vi "Do_Every_minute.vi"(1 "Ch Names":string[](array[string]), 2 "Values":dbl[](array[numeric]) format="%.2f") -> (0 "Scan Comments":string)   [LabVIEW 2022 SP3]
uses:
  Anemometry/Anemometry Sub Vis/Controls/In_Range.ctl
  ADAM Client/Sub VIs/ADAM Controls/Update_scan_value.ctl
  ADAM Client/Sub VIs/Channel_State_Control.ctl
  ADAM Client/Sub VIs/ADAM Controls/Traverse_Level_State.ctl
  Anemometry/Anemometry Sub Vis/Globals/EnFlo_Tunnel_Global.vi
  Anemometry/Anemometry Sub Vis/Globals/Gas_management_global.vi
  ADAM_Global.vi
panel:
  in  "Kp":dbl=50.0 format="%#_13g"
  in  "Deadband Delta T":dbl=0.002 format="%#_13g"
  out "Max Delta T":dbl(graph)
  in  "Manual Control of Lamps":bool
  out "Power":dbl[][](graph)=[[0.00729, 0.18153463174730816, 0.17352738437348433, 1.6752433719500537, 8.231465735195274, 17.570357598383207, 23.099772817121426, 25.58386930448374, 25.31727725753219, 24.28926231541072, 18.717383219374323, 10.355253339797807, 2.7760273383248344, 0.3109897541921306, 0.08276881403435009, 0.06197], [0.04411, 0.1361526368018142, 0.04039202183336771, 1.5611636795339547, 8.176972694107874, 17.32000974741714, 24.257541358764026, 25.949153465972987, 26.01802540761648, 25.060373307424115, 18.284750328365213, 8.689831176707928, 2.642937641487066, 0.43219350072447926, -0.019957690739617468, 0.07351], [0.05478, 0.03446320268089581, 0.2086595806581808, 1.6919212249796047, 6.580368005180591, 14.333585185483123, 21.06810094963999, 23.709254571137723, 24.04768940379576, 21.01660820522005, 13.60443428327954, 6.2766496258038735, 1.7988963349022484, 0.2952877651784204, 0.05436788410934033, 0.1022], [0.04013, 0.06419557464541133, 0.2035068586120256, 1.3118741659450193, 4.7061387064566835, 9.009825946069038, 12.927700276268434, 17.003135081884164, 16.83885730812343, 12.902263313363814, 8.246161922417906, 4.035269404379355, 1.329605659745338, 0.24574055091433544, 0.012829784119986217, 0.08755], [0.04404, 0.022691144295571734, 0.19102098261858932, 0.8525411026079828, 2.2353542219792946, 3.966676465246214, 6.305347763088489, 8.17672908183636, 7.7348668140659, 5.703994479070454, 3.8329088824353237, 1.9256956625267279, 0.6611488869641811, 0.20508248283573002, 0.10119553469307395, 0.08441]]
  out "Temperature":dbl[][](graph)=[[0.00729, 0.18153463174730816, 0.17352738437348433, 1.6752433719500537, 8.231465735195274, 17.570357598383207, 23.099772817121426, 25.58386930448374, 25.31727725753219, 24.28926231541072, 18.717383219374323, 10.355253339797807, 2.7760273383248344, 0.3109897541921306, 0.08276881403435009, 0.06197], [0.04411, 0.1361526368018142, 0.04039202183336771, 1.5611636795339547, 8.176972694107874, 17.32000974741714, 24.257541358764026, 25.949153465972987, 26.01802540761648, 25.060373307424115, 18.284750328365213, 8.689831176707928, 2.642937641487066, 0.43219350072447926, -0.019957690739617468, 0.07351], [0.05478, 0.03446320268089581, 0.2086595806581808, 1.6919212249796047, 6.580368005180591, 14.333585185483123, 21.06810094963999, 23.709254571137723, 24.04768940379576, 21.01660820522005, 13.60443428327954, 6.2766496258038735, 1.7988963349022484, 0.2952877651784204, 0.05436788410934033, 0.1022], [0.04013, 0.06419557464541133, 0.2035068586120256, 1.3118741659450193, 4.7061387064566835, 9.009825946069038, 12.927700276268434, 17.003135081884164, 16.83885730812343, 12.902263313363814, 8.246161922417906, 4.035269404379355, 1.329605659745338, 0.24574055091433544, 0.012829784119986217, 0.08755], [0.04404, 0.022691144295571734, 0.19102098261858932, 0.8525411026079828, 2.2353542219792946, 3.966676465246214, 6.305347763088489, 8.17672908183636, 7.7348668140659, 5.703994479070454, 3.8329088824353237, 1.9256956625267279, 0.6611488869641811, 0.20508248283573002, 0.10119553469307395, 0.08441]]
  in  "Kp Lamps":dbl=50.0 format="%#_13g"
  in  "Averaging time in Seconds":dbl=200.0 format="%#_13g"
  in  "Disable Sending email to estates regarding Chilled water Temp":bool=TRUE
  in  "Max K Factor":dbl=16.0
  # "Control Parameters"
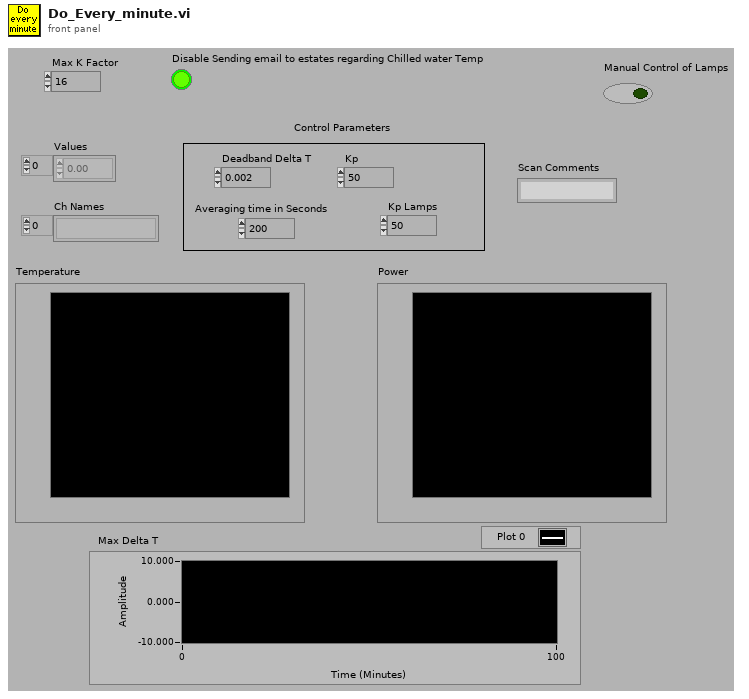
[diagram p1: front panel]
types:
  T1 = typedef "In_Range.ctl" = enum16{"%", "±", "% & ±"}
  T2 = typedef "Update_scan_value.ctl" = cluster{"Channel Name":string, "New Value":dbl, "!Auto_Off":bool}
  T3 = enum16{"Append to Global", "Read Global then Clear"}
  T4 = typedef "Channel_State_Control.ctl" = enum16{"Channel Name", "Channel Name Starts with", "Main Address"}
  T5 = typedef "Traverse_Level_State.ctl" = enum16{"Running", "Complete"}
  T6 = typedef "Ch_description_ADAM.ctl" = cluster{"Ch Name":string, "Type":T7, "Function":T8, "Ch State":T9, "Calibration type":T10, "A":dbl, "B":dbl, "C":dbl, "D":dbl, "Comments":string, "Address":T11, "String":string, "Duty":u16}
  T7 = typedef "Module_type_ADAM.ctl" = string
  T8 = typedef "Function_ADAM.ctl" = enum16{"Analogue Input", "Digital Input", "Event counter", "Event rate", "Analogue Output", "Digital Output", "Relay Output"}
  T9 = typedef "Channel_State.ctl" = enum16{"On", "Off", "Always On", "Always Off"}
  T10 = typedef "Calib_type_ADAM.ctl" = string
  T11 = typedef "Address.ctl" = cluster{"Main":i32, "Ch.":i32, "Sub":i32, "Port Name":string}
  T12 = cluster{"Bus Bar":string, "Connected Items":string[]}
  T13 = cluster{"Ch Name":string, "subarray":string[], "subarray":dbl[], i32, i32}
  T14 = typedef "Client_State_Cluster.ctl" = cluster{"Client Name":string, "Traverse level State":T5, "People to Email":string[], "Next Contact Time":dbl}
  T15 = cluster{"second":i32, "minute":i32, "hour":i32, "day of month":i32, "month":i32, "year":i32, "day of week":i32, "day of year":i32, "is DST":i32}
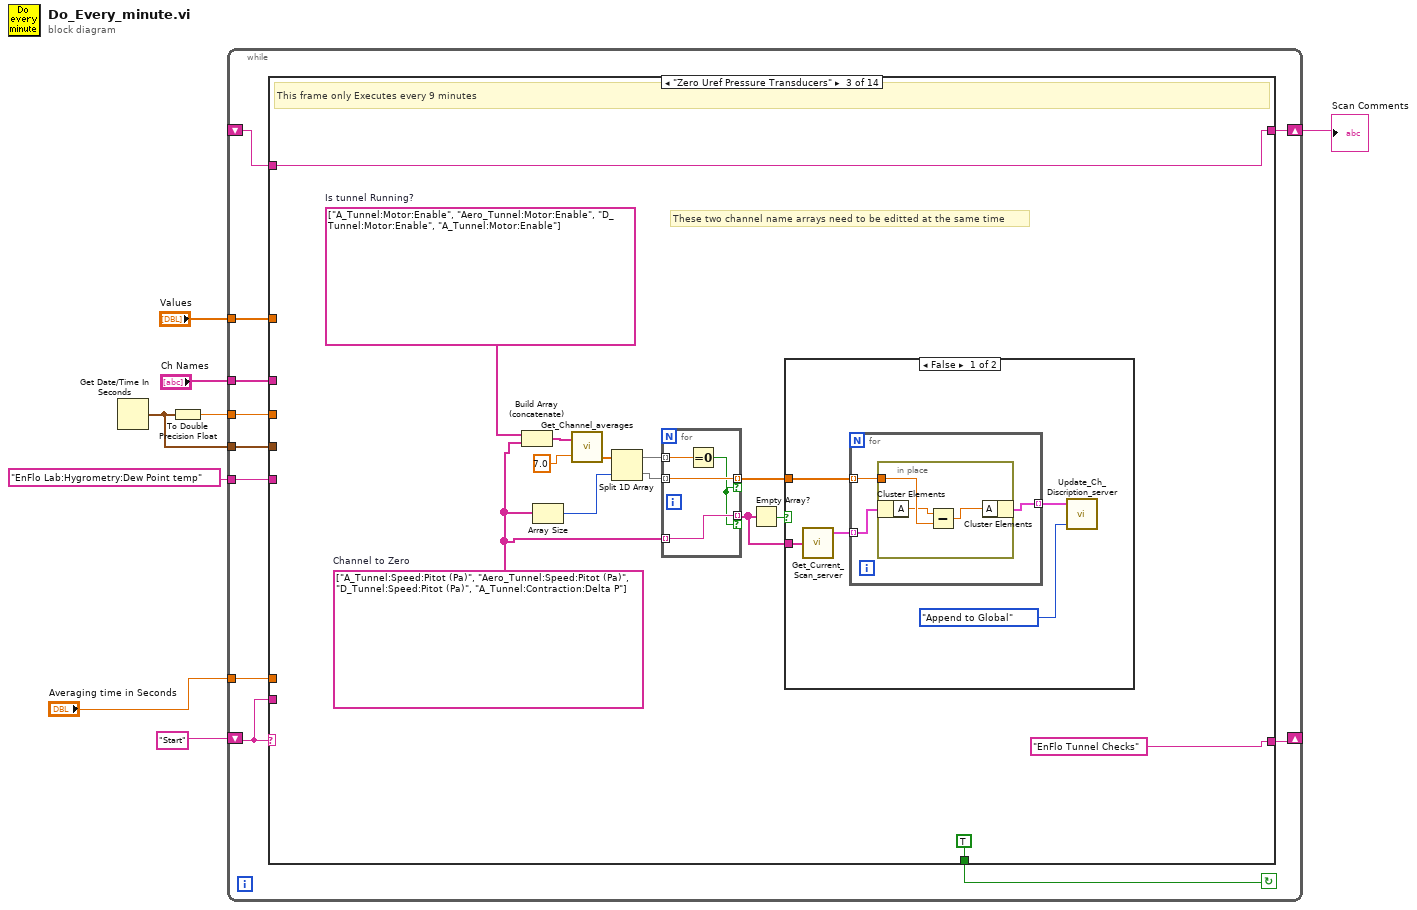
[diagram p0: block diagram]
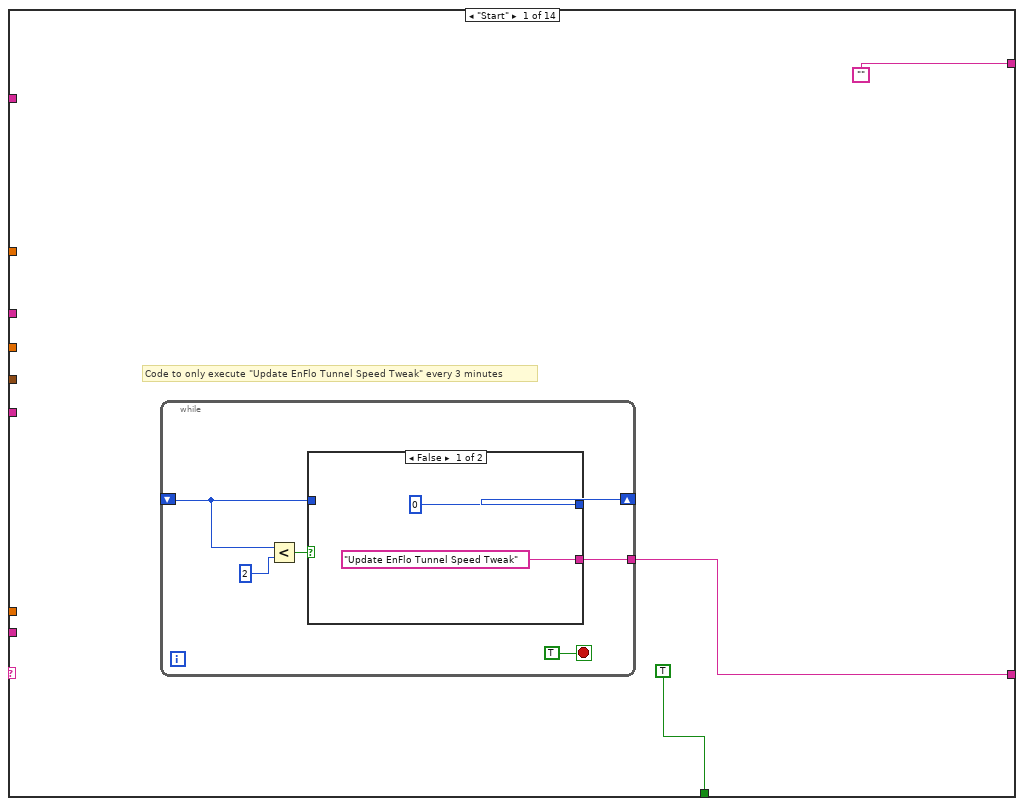
[diagram p2: hidden frame]
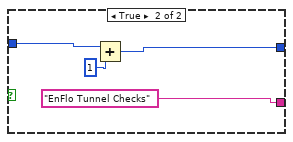
[diagram p3: hidden frame]
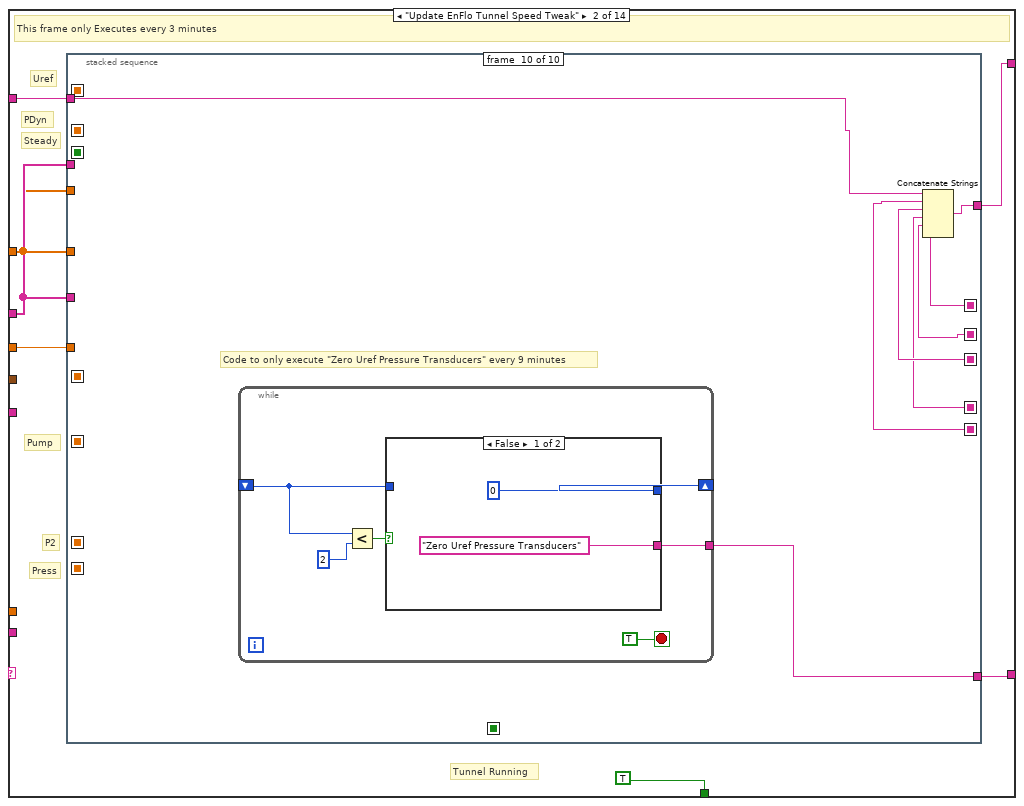
[diagram p4: hidden frame]
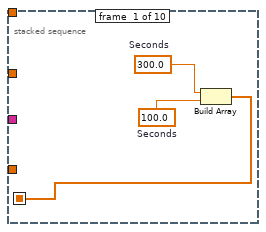
[diagram p5: hidden frame]
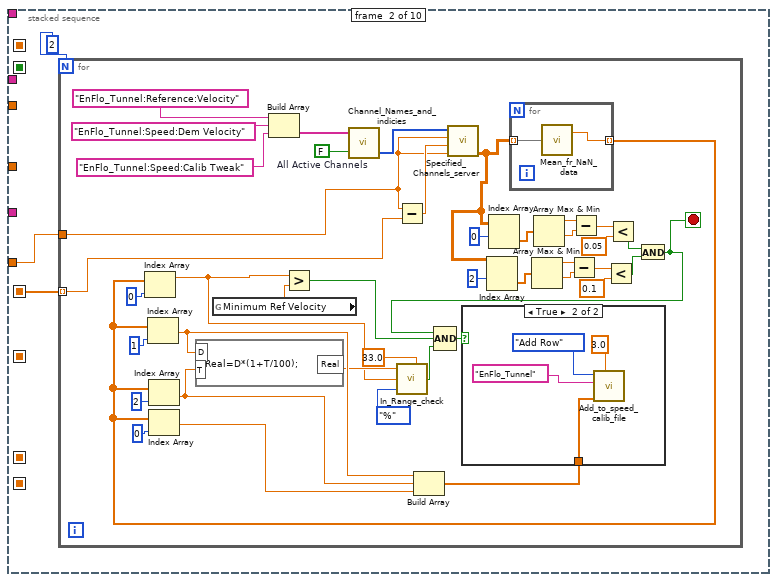
[diagram p6: hidden frame]
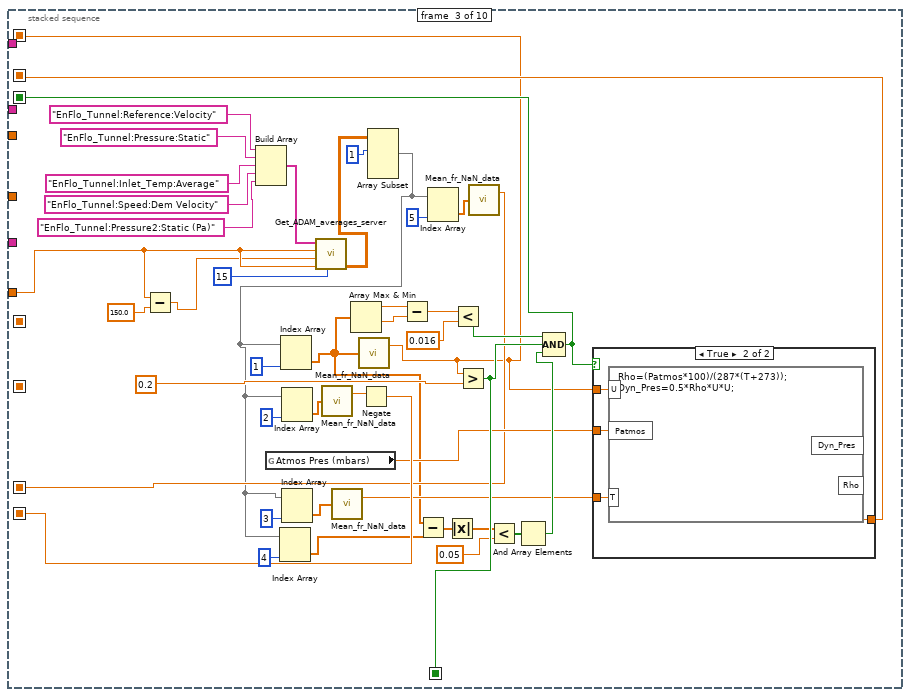
[diagram p8: hidden frame]
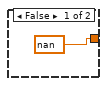
[diagram p9: hidden frame]
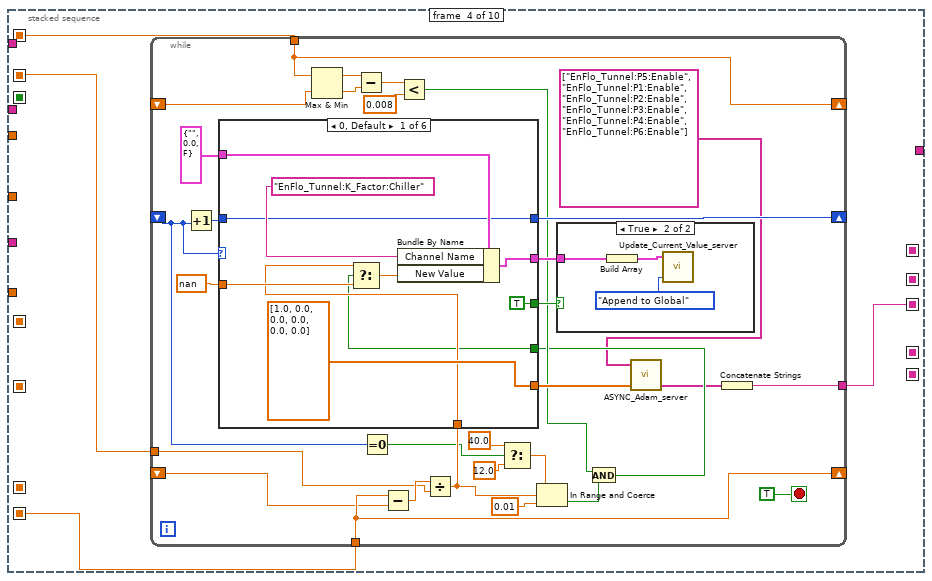
[diagram p10: hidden frame]
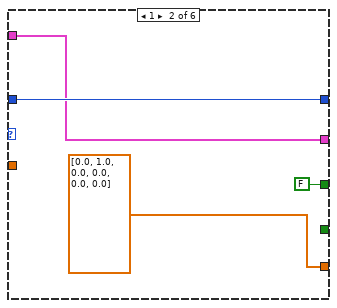
[diagram p12: hidden frame]
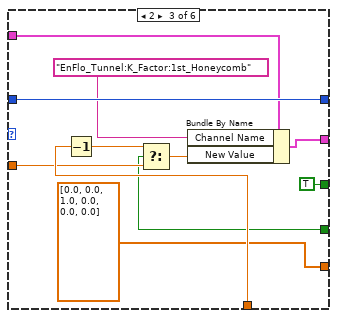
[diagram p13: hidden frame]
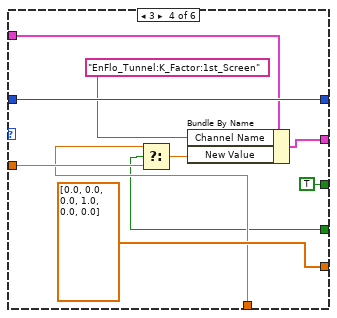
[diagram p14: hidden frame]
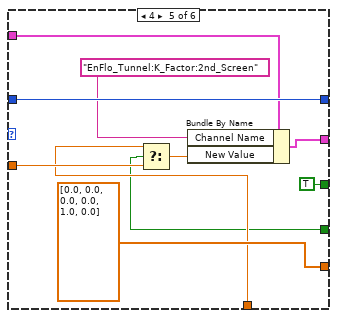
[diagram p15: hidden frame]
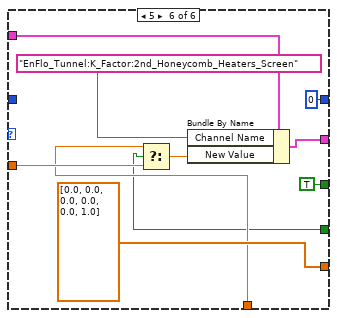
[diagram p16: hidden frame]
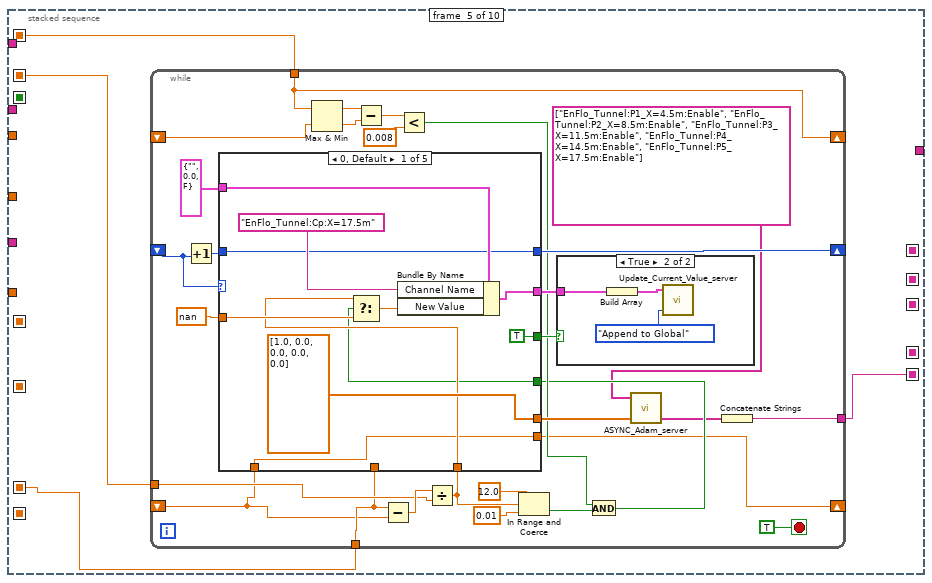
[diagram p17: hidden frame]
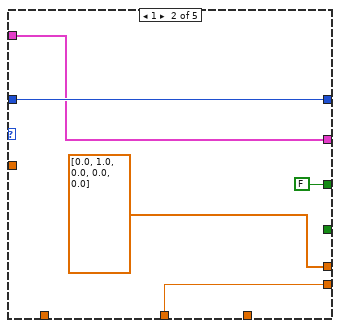
[diagram p19: hidden frame]
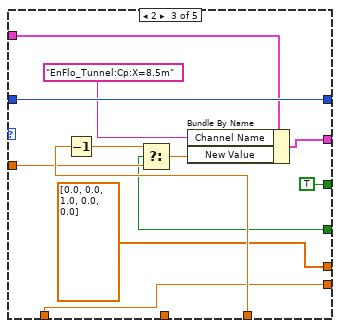
[diagram p20: hidden frame]
diagram:
  n1 = Get Date/Time In Seconds() -> (seconds since 1Jan1904=w4:timestamp)
  n2 = To Double Precision Float(number=w4) -> (double precision float=w5:dbl)
  n3 = while {
    tunnel: "EnFlo Lab:Hygrometry:Dew Point temp" -> [w15]
    tunnel: "Values" -> [w17]
    tunnel: "Ch Names" -> [w18]
    shift-left: "Start" -> [w12]
    shift-right: [w16] -> _
    tunnel: w5 -> [w14]
    tunnel: w4 -> [w13]
    tunnel: "Averaging time in Seconds" -> [w11]
    shift-right: [w10] -> w1
    shift-left: _ -> [w9]
    stop <- w19 continue-if-true
    n4 = case shown="\"Zero Uref Pressure Transducers\"" w12 {
      tunnel: [TRUE TRUE TRUE TRUE TRUE TRUE TRUE TRUE TRUE TRUE TRUE TRUE FALSE FALSE] -> w19
      tunnel: w18 -> [_ w37 _ w530 w725 _ _ _ w1013 w1040 w1076 w1116 w1128 _]
      tunnel: w17 -> [_ w36 _ w531 w726 _ _ _ w1014 w1041 w1077 w1117 w1127 _]
      tunnel: [w21 w35 "EnFlo Tunnel Checks" w529 w724 w953 "Lab Temp Control" "Is Dew point meter Alive?" w1017 w1028 "More checks" "End" "End" "End"] -> w16
      tunnel: w15 -> [_ _ _ _ _ _ _ _ w1012 _ _ _ _ _]
      tunnel: w14 -> [_ w40 _ w528 w728 _ _ w991 _ _ _ _ w1126 _]
      tunnel: w13 -> [_ _ _ _ _ _ _ _ _ _ _ _ w1129 _]
      tunnel: w12 -> [_ _ _ _ _ _ _ _ _ _ _ _ _ w1196]
      tunnel: w11 -> [_ _ _ w527 w727 _ _ _ _ _ _ _ _ _]
      tunnel: ["" w38 w497 w525 w722 w951 w966 w990 w994 w1026 w1065 w1112 w1122 w1193] -> w10
      tunnel: w9 -> [_ w39 w497 w526 w723 w951 w966 w990 w996 w1027 w1066 w1113 w1123 w1193]
      frame "Start" {
        # "Code to only execute \"Update EnFlo Tunnel Speed Tweak\" every 3 minutes"
        n5 = while {
          shift-right: [w25] -> _
          shift-left: _ -> [w23]
          tunnel: [w24] -> w21
          stop <- TRUE stop-if-true
          n6 = Less?(x=w23, y=2) -> (x < y?=w26:bool)
          n7 = case shown="False" w26 {
            tunnel: [0 w32] -> w25
            tunnel: ["Update EnFlo Tunnel Speed Tweak" "EnFlo Tunnel Checks"] -> w24
            tunnel: w23 -> [_ w33]
            frame False {
            }
            frame True {
              n8 = Add(x=w33, y=1) -> (x+y=w32:i32)
            }
          }
        }
      }
      frame "Update EnFlo Tunnel Speed Tweak" {
        # "P2"
        # "Pump"
        # "Tunnel Running"
        # "PDyn"
        # "Steady"
        # "Press"
        # "Uref"
        # "This frame only Executes every 3 minutes"
        n9 = stacked-sequence {
          seq-local: [w42 _ _ _ _ _ _ _ _ _] -> [_ w46 _ _ _ _ _ _ _ _]
          seq-local: [_ _ w99 _ _ _ _ _ _ _] -> [_ _ _ w145 w240 _ _ _ _ _]
          seq-local: [_ _ w123 _ _ _ _ _ _ _] -> [_ _ _ w147 _ _ _ _ _ _]
          seq-local: [_ _ w121 _ _ _ _ _ _ _] -> [_ _ _ _ _ _ _ _ _ _]
          seq-local: [_ _ w124 _ _ _ _ _ _ _] -> [_ _ _ w146 w238 _ _ _ _ _]
          seq-local: [_ _ w120 _ _ _ _ _ _ _] -> [_ _ _ _ _ _ _ w384 _ _]
          seq-local: [_ _ _ w144 _ _ _ _ _ _] -> [_ _ _ _ _ _ _ _ _ w482]
          seq-local: [_ _ _ _ _ w324 _ _ _ _] -> [_ _ _ _ _ _ w332 _ _ _]
          seq-local: [_ _ _ _ _ w323 _ _ _ _] -> [_ _ _ _ _ _ _ _ _ w480]
          seq-local: [_ _ _ _ _ _ w328 _ _ _] -> [_ _ _ _ _ _ _ _ _ w479]
          seq-local: [_ _ _ _ _ _ _ w383 _ _] -> [_ _ _ _ _ _ _ _ _ w478]
          seq-local: [_ _ w105 _ _ _ _ _ _ _] -> [_ _ _ _ w237 _ _ _ _ _]
          seq-local: [_ _ _ _ w239 _ _ _ _ _] -> [_ _ _ _ _ _ _ _ _ w477]
          tunnel: w37 -> [_ _ _ _ _ w326 w329 _ _ _]
          tunnel: w36 -> [_ _ _ _ _ w327 w330 _ _ _]
          tunnel: w40 -> [_ w45 w138 _ _ _ _ w382 _ _]
          tunnel: w39 -> [_ _ _ _ _ _ _ _ _ w483]
          tunnel: [_ _ _ _ _ _ _ _ _ w481] -> w38
          tunnel: w37 -> [_ _ _ _ _ _ _ _ _ _]
          tunnel: w36 -> [_ _ _ _ _ _ _ _ _ _]
          tunnel: [_ _ _ _ _ _ _ _ _ w476] -> w35
          frame #0 {
            w43 = 100.0  # Seconds
            w44 = 300.0  # Seconds
            n10 = Build Array(w44, w43) -> (w42:dbl[])
          }
          frame #1 {
            n11 = for {
              N: 2 -> [_]
              tunnel: w45 -> [w51]
              tunnel: w46 -> [w50] mode=indexing
              stop <- w49 stop-if-true
              w81 = FALSE  # All Active Channels
              n12 = global read "EnFlo_Tunnel_Global.vi" "Minimum Ref Velocity"() -> (w48:dbl)
              n13 = Build Array("EnFlo_Tunnel:Reference:Velocity", "EnFlo_Tunnel:Speed:Dem Velocity", "EnFlo_Tunnel:Speed:Calib Tweak") -> (w79:string[])
              n14 = call "Channel_Names_and_indicies.vi"("All Active Channels"=w81, "Desired Ch Names"=w79) -> ("Indicies"=w80:i32[])  [unwired: 1 out]
              n15 = Subtract(x=w51, y=w50) -> (x-y=w78:dbl)
              n16 = call "Specified_Channels_server.vi"("End time"=w51, "Start time"=w78, "Clients time"=w51, "Requested channels"=w80) -> ("Output array"=w61:dbl[][])  [unwired: 1 in, 4 out]
              n17 = Index Array(array=w61, index (row)=2 ("Index")) -> (element=w63:dbl[])  [unwired: 1 in]
              n18 = Index Array(array=w61, index (row)=0 ("Index")) -> (element=w76:dbl[])  [unwired: 1 in]
              n19 = for {
                tunnel: w61 -> [w91] mode=indexing
                tunnel: [w90] -> w69 mode=indexing
                n20 = call "Mean_fr_NaN_data.vi"("Data"=w91) -> ("Mean value"=w90:dbl)  [unwired: 1 out]
              }
              n21 = Index Array(array=w69, index=0) -> (element=w55:dbl)
              n22 = Index Array(array=w69, index=1) -> (element=w57:dbl)
              n23 = Index Array(array=w69, index=2) -> (element=w58:dbl)
              n24 = Index Array(array=w69, index=0) -> (element=w68:dbl)
              n25 = formula code="Real=D*(1+T/100);"("D"=w57, "T"=w58) -> ("Real"=w56:dbl)
              n26 = Greater?(x=w55, y=w48) -> (0:w84:bool)
              n27 = call "In_Range_check.vi"("%"=33.0, "Mode"=In_Range."%", "Value"=w55, "Setpoint"=w56) -> ("In Range"=w52:bool)  [unwired: 1 in, 2 out]
              n28 = Build Array(w57, w58, w68) -> (w83:dbl[])
              n29 = Array Max & Min(array=w63) -> (max value=w64:dbl, min value=w65:dbl)  [unwired: 2 out]
              n30 = Array Max & Min(array=w76) -> (max value=w75:dbl, min value=w74:dbl)  [unwired: 2 out]
              n31 = Subtract(x=w64, y=w65) -> (x-y=w66:dbl)
              n32 = Subtract(x=w75, y=w74) -> (x-y=w73:dbl)
              n33 = Less?(x=w66, y=0.1) -> (x < y?=w60:bool)
              n34 = Less?(x=w73, y=0.05) -> (x < y?=w59:bool)
              n35 = And(x=w59, y=w60) -> (x .and. y?=w49:bool)
              n36 = Compound Arithmetic op=AND(w49, w84, w52) -> (w82:bool)
              n37 = case shown="True" w82 {
                tunnel: w83 -> [_ w94]
                frame False {
                }
                frame True {
                  n38 = call "Add_to_speed_calib_file.vi"("Max Velocity"=3.0, "New Row"=w94, "Rig Name"="EnFlo_Tunnel" ("y"), "Mode"=enum16{"Add Row", "Get Error Value"}."Add Row") -> ()  [unwired: 2 in, 2 out]
                }
              }
            }
          }
          frame #2 {
            n39 = Subtract(x=w138, y=150.0) -> (x-y=w136:dbl)
            n40 = Build Array("EnFlo_Tunnel:Reference:Velocity", "EnFlo_Tunnel:Pressure:Static", "EnFlo_Tunnel:Inlet_Temp:Average", "EnFlo_Tunnel:Speed:Dem Velocity", "EnFlo_Tunnel:Pressure2:Static (Pa)") -> (w135:string[])
            n41 = global read "Gas_management_global.vi" "Atmos Pres (mbars)"() -> (w107:dbl)
            n42 = call "Get_ADAM_averages_server.vi"("No of averages"=15, "End time"=w138, "Start time"=w136, "Clients time"=w138, "ADAM Ch Names"=w135) -> ("DBL values"=w98:dbl[][])  [unwired: 1 in, 4 out]
            n43 = Array Subset(array=w98, index (row)=1 ("index")) -> (w96:dbl[][])  [unwired: 3 in]
            n44 = Index Array(array=w96, index (col)=4 ("disabled index (col)")) -> (element=w113:dbl[])  [unwired: 1 in]
            n45 = Index Array(array=w96, index (col)=1 ("disabled index (col)")) -> (element=w100:dbl[])  [unwired: 1 in]
            n46 = Index Array(array=w96, index (col)=2 ("disabled index (col)")) -> (element=w102:dbl[])  [unwired: 1 in]
            n47 = Index Array(array=w96, index (col)=3 ("disabled index (col)")) -> (element=w104:dbl[])  [unwired: 1 in]
            n48 = call "Mean_fr_NaN_data.vi"("Data"=w102) -> ("Mean value"=w101:dbl)  [unwired: 1 out]
            n49 = call "Mean_fr_NaN_data.vi"("Data"=w104) -> ("Mean value"=w103:dbl)  [unwired: 1 out]
            n50 = Array Max & Min(array=w100) -> (max value=w130:dbl, min value=w131:dbl)  [unwired: 2 out]
            n51 = call "Mean_fr_NaN_data.vi"("Data"=w100) -> ("Mean value"=w99:dbl)  [unwired: 1 out]
            n52 = Negate(x=w101) -> (-x=w123:dbl)
            n53 = Subtract(x=w130, y=w131) -> (x-y=w132:dbl)
            n54 = Subtract(x=w100, y=w113) -> (x-y=w116:dbl[])
            n55 = Index Array(array=w96, index (col)=5 ("disabled index (col)")) -> (element=w106:dbl[])  [unwired: 1 in]
            n56 = Absolute Value(x=w116) -> (abs(x)=w115:dbl[])
            n57 = Less?(x=w132, y=0.016) -> (x < y?=w122:bool)
            n58 = Greater?(x=w99, y=0.2) -> (0:w120:bool)
            n59 = call "Mean_fr_NaN_data.vi"("Data"=w106) -> ("Mean value"=w105:dbl)  [unwired: 1 out]
            n60 = Less?(x=w115, y=0.05) -> (x < y?=w112:bool[])
            n61 = And Array Elements(Boolean array=w112) -> (logical AND=w111:bool)
            n62 = Compound Arithmetic op=AND(w122, w120, w111) -> (w121:bool)
            n63 = case shown="True" w121 {
              tunnel: w103 -> [_ w143]
              tunnel: w107 -> [_ w142]
              tunnel: w99 -> [_ w141]
              tunnel: [nan w140] -> w124
              frame False {
              }
              frame True {
                n64 = formula code="Rho=(Patmos*100)/(287*(T+273));\nDyn_Pres=0.5*Rho*U*U;"("Patmos"=w142, "T"=w143, "U"=w141) -> ("Dyn_Pres"=w140:dbl)  [unwired: 1 out]
              }
            }
          }
          frame #3 {
            n65 = while {
              shift-right: [w177] -> _
              shift-left: _ -> [w152]
              shift-right: [w174] -> _
              shift-left: _ -> [w173]
              tunnel: w147 -> [w174]
              tunnel: w146 -> [w171]
              shift-right: [w170] -> _
              shift-left: _ -> [w169]
              tunnel: w145 -> [w170]
              tunnel: [w154] -> w144
              stop <- TRUE stop-if-true
              n66 = Increment(x=w152) -> (x+1=w176:i32)
              n67 = Max & Min(x=w170, y=w169) -> (max(x,y)=w168:dbl, min(x,y)=w167:dbl)
              n68 = Subtract(x=w168, y=w167) -> (x-y=w166:dbl)
              n69 = Equal To 0?(x=w152) -> (x = 0?=w150:bool)
              n70 = Subtract(x=w174, y=w173) -> (x-y=w172:dbl)
              n71 = Less?(x=w166, y=0.008) -> (x < y?=w157:bool)
              n72 = Divide(x=w172, y=w171) -> (x/y=w160:dbl)
              n73 = Select(t=40.0 ("upper limit"), s=w150, f=12.0) -> (s? t:f=w149:dbl)
              n74 = In Range and Coerce(upper limit=w149, x=w160, lower limit=0.01) -> (In Range?=w158:bool)  [unwired: 1 out]
              n75 = And(x=w157, y=w158) -> (x .and. y?=w156:bool)
              n76 = case shown="0, Default" w152 {
                tunnel: [w184 w195 w206 w216 w226 0] -> w177
                tunnel: w176 -> [w184 w195 w206 w216 w226 _]
                tunnel: T2 {"Channel Name"="", "New Value"=0.0, "!Auto_Off"=FALSE} ("Update Scan Value Cluster") -> [w191 w194 w205 w215 w225 w236]
                tunnel: w160 -> [w185 _ w203 w209 w219 w230]
                tunnel: [w189 w194 w202 w213 w223 w234] -> w164
                tunnel: nan -> [w188 _ w200 w212 w222 w233]
                tunnel: [dbl[] [1.0, 0.0, 0.0, 0.0, 0.0, 0.0] ("Values") dbl[] [0.0, 1.0, 0.0, 0.0, 0.0, 0.0] ("Values") dbl[] [0.0, 0.0, 1.0, 0.0, 0.0, 0.0] ("Values") dbl[] [0.0, 0.0, 0.0, 1.0, 0.0, 0.0] ("Values") dbl[] [0.0, 0.0, 0.0, 0.0, 1.0, 0.0] ("Values") dbl[] [0.0, 0.0, 0.0, 0.0, 0.0, 1.0] ("Values")] -> w162
                tunnel: [TRUE FALSE TRUE TRUE TRUE TRUE] -> w161
                tunnel: w156 -> [w182 _ w196 w207 w217 w227]
                frame 0, Default {
                  n77 = Select(t=w185, s=w182, f=w188) -> (s? t:f=w187:dbl)
                  n78 = Bundle By Name(cluster=w191, "Channel Name"="EnFlo_Tunnel:K_Factor:Chiller", "New Value"=w187) -> (w189:T2)
                }
                frame 1 {
                }
                frame 2 {
                  n79 = Decrement(x=w203) -> (x-1=w201:dbl)
                  n80 = Select(t=w201, s=w196, f=w200) -> (s? t:f=w199:dbl)
                  n81 = Bundle By Name(cluster=w205, "Channel Name"="EnFlo_Tunnel:K_Factor:1st_Honeycomb", "New Value"=w199) -> (w202:T2)
                }
                frame 3 {
                  n82 = Select(t=w209, s=w207, f=w212) -> (s? t:f=w211:dbl)
                  n83 = Bundle By Name(cluster=w215, "Channel Name"="EnFlo_Tunnel:K_Factor:1st_Screen", "New Value"=w211) -> (w213:T2)
                }
                frame 4 {
                  n84 = Select(t=w219, s=w217, f=w222) -> (s? t:f=w221:dbl)
                  n85 = Bundle By Name(cluster=w225, "Channel Name"="EnFlo_Tunnel:K_Factor:2nd_Screen", "New Value"=w221) -> (w223:T2)
                }
                frame 5 {
                  n86 = Select(t=w230, s=w227, f=w233) -> (s? t:f=w232:dbl)
                  n87 = Bundle By Name(cluster=w236, "Channel Name"="EnFlo_Tunnel:K_Factor:2nd_Honeycomb_Heaters_Screen", "New Value"=w232) -> (w234:T2)
                }
              }
              n88 = case shown="True" w161 {
                tunnel: w164 -> [_ w179]
                frame False {
                }
                frame True {
                  n89 = Build Array(w179) -> (w180:T2[])
                  n90 = call "Update_Current_Value_server.vi"("Mode"=T3."Append to Global", "Update array in"=w180) -> ()  [unwired: 1 in, 1 out]
                }
              }
              n91 = call "ASYNC_Adam_server.vi"("Values"=w162, "Channel Names"=string[] ["EnFlo_Tunnel:P5:Enable", "EnFlo_Tunnel:P1:Enable", "EnFlo_Tunnel:P2:Enable", "EnFlo_Tunnel:P3:Enable", "EnFlo_Tunnel:P4:Enable", "EnFlo_Tunnel:P6:Enable"]) -> ("Scan Comments"=w155:string[])  [unwired: 1 in, 2 out]
              n92 = Concatenate Strings(w155) -> (w154:string)
            }
          }
          frame #4 {
            n93 = while {
              shift-right: [w268] -> _
              shift-left: _ -> [w266]
              shift-right: [w244] -> _
              shift-left: _ -> [w242]
              tunnel: w237 -> [w243]
              tunnel: w238 -> [w263]
              shift-right: [w262] -> _
              shift-left: _ -> [w261]
              tunnel: w240 -> [w262]
              tunnel: [w245] -> w239
              stop <- TRUE stop-if-true
              n94 = Increment(x=w266) -> (x+1=w267:i32)
              n95 = Max & Min(x=w262, y=w261) -> (max(x,y)=w260:dbl, min(x,y)=w259:dbl)
              n96 = Subtract(x=w260, y=w259) -> (x-y=w258:dbl)
              n97 = Subtract(x=w243, y=w242) -> (x-y=w264:dbl)
              n98 = Less?(x=w258, y=0.008) -> (x < y?=w248:bool)
              n99 = Divide(x=w264, y=w263) -> (x/y=w252:dbl)
              n100 = In Range and Coerce(upper limit=12.0, x=w252, lower limit=0.01) -> (In Range?=w249:bool)  [unwired: 1 out]
              n101 = And(x=w248, y=w249) -> (x .and. y?=w247:bool)
              n102 = case shown="0, Default" w266 {
                tunnel: [w276 w288 w300 w311 0] -> w268
                tunnel: w267 -> [w276 w288 w300 w311 _]
                tunnel: T2 {"Channel Name"="", "New Value"=0.0, "!Auto_Off"=FALSE} ("Update Scan Value Cluster") -> [w283 w287 w299 w310 w322]
                tunnel: w252 -> [w277 _ w297 w304 w316]
                tunnel: [w281 w287 w296 w308 w320] -> w256
                tunnel: nan -> [w280 _ w294 w307 w319]
                tunnel: [dbl[] [1.0, 0.0, 0.0, 0.0, 0.0] ("Values") dbl[] [0.0, 1.0, 0.0, 0.0, 0.0] ("Values") dbl[] [0.0, 0.0, 1.0, 0.0, 0.0] ("Values") dbl[] [0.0, 0.0, 0.0, 1.0, 0.0] ("Values") dbl[] [0.0, 0.0, 0.0, 0.0, 1.0] ("Values")] -> w254
                tunnel: [TRUE FALSE TRUE TRUE TRUE] -> w253
                tunnel: w247 -> [w274 _ w290 w302 w313]
                tunnel: [w273 w284 w289 w301 w312] -> w244
                tunnel: w243 -> [_ w284 _ _ _]
                tunnel: w242 -> [w273 _ w289 w301 w312]
                frame 0, Default {
                  n103 = Select(t=w277, s=w274, f=w280) -> (s? t:f=w279:dbl)
                  n104 = Bundle By Name(cluster=w283, "Channel Name"="EnFlo_Tunnel:Cp:X=17.5m", "New Value"=w279) -> (w281:T2)
                }
                frame 1 {
                }
                frame 2 {
                  n105 = Decrement(x=w297) -> (x-1=w295:dbl)
                  n106 = Select(t=w295, s=w290, f=w294) -> (s? t:f=w293:dbl)
                  n107 = Bundle By Name(cluster=w299, "Channel Name"="EnFlo_Tunnel:Cp:X=8.5m", "New Value"=w293) -> (w296:T2)
                }
                frame 3 {
                  n108 = Select(t=w304, s=w302, f=w307) -> (s? t:f=w306:dbl)
                  n109 = Bundle By Name(cluster=w310, "Channel Name"="EnFlo_Tunnel:Cp:X=11.5m", "New Value"=w306) -> (w308:T2)
                }
                frame 4 {
                  n110 = Select(t=w316, s=w313, f=w319) -> (s? t:f=w318:dbl)
                  n111 = Bundle By Name(cluster=w322, "Channel Name"="EnFlo_Tunnel:Cp:X=14.5m", "New Value"=w318) -> (w320:T2)
                }
              }
              n112 = case shown="True" w253 {
                tunnel: w256 -> [_ w270]
                frame False {
                }
                frame True {
                  n113 = Build Array(w270) -> (w271:T2[])
                  n114 = call "Update_Current_Value_server.vi"("Mode"=T3."Append to Global", "Update array in"=w271) -> ()  [unwired: 1 in, 1 out]
                }
              }
              n115 = call "ASYNC_Adam_server.vi"("Values"=w254, "Channel Names"=string[] ["EnFlo_Tunnel:P1_X=4.5m:Enable", "EnFlo_Tunnel:P2_X=8.5m:Enable", "EnFlo_Tunnel:P3_X=11.5m:Enable", "EnFlo_Tunnel:P4_X=14.5m:Enable", "EnFlo_Tunnel:P5_X=17.5m:Enable"]) -> ("Scan Comments"=w246:string[])  [unwired: 1 in, 2 out]
              n116 = Concatenate Strings(w246) -> (w245:string)
            }
          }
          frame #5 {
            n117 = call "Read_value_of_earlier_Ch.vi"("Desired Ch to Read"="EnFlo_Tunnel:Chiller_Pump:Running", "Ch names"=w326, "Present scan array"=w327) -> ("Value"=w324:dbl, "Scan comment"=w323:string)  [unwired: 1 in]
          }
          frame #6 {
            n118 = Greater?(x=w332, y=0.5) -> (0:w331:bool)
            n119 = case shown="True" w331 {
              tunnel: w330 -> [_ w355]
              tunnel: w329 -> [_ w354]
              tunnel: ["" w345] -> w328
              frame False {
              }
              frame True {
                w348 = errorcluster {"status"=FALSE, "code"=0, "source"=""} ("error in (no error)")
                w347 = string[] ["EnFlo_Tunnel:Power:Chiller_Pump_Exchanger", "EnFlo_Tunnel:Meas Power:Chiller_Pump_Exchanger", "EnFlo_Tunnel:Power:Chiller_Pump_Floor", "EnFlo_Tunnel:Meas Power:Chiller_Pump_Floor"]
                n120 = call "Read_Earlier_Channels.vi"("Present scan array"=w355, "Ch names"=w354, "Desired Channels"=w347) -> ("Scan comments"=w345:string, "Index 0"=w344:dbl, "Index 1"=w349:dbl, "Index 2"=w339:dbl, "Index 3"=w346:dbl)  [unwired: 1 out]
                n121 = feedback-in #1(w344) -> ()
                n122 = feedback #1() -> (w343:dbl)  [unwired: 1 in]
                n123 = Equal?(x=w343, y=w344) -> (x = y?=w342:bool)
                n124 = call "In_Range_check.vi"("±"=6.0, "Mode"=In_Range."±", "Value"=w346, "Setpoint"=w339) -> ("In Range"=w336:bool)  [unwired: 3 in]
                n125 = call "In_Range_check.vi"("±"=6.0, "Mode"=In_Range."±", "Value"=w349, "Setpoint"=w344) -> ("In Range"=w341:bool)  [unwired: 3 in]
                n126 = feedback #2() -> (w338:dbl)  [unwired: 1 in]
                n127 = feedback-in #2(w339) -> ()
                n128 = Compound Arithmetic op=AND(w342, invert w341) -> (w340:bool)
                n129 = Equal?(x=w339, y=w338) -> (x = y?=w337:bool)
                n130 = Compound Arithmetic op=AND(w337, invert w336) -> (w335:bool)
                n131 = case shown="True" w340 {
                  tunnel: w348 -> [_ _]
                  tunnel: w347 -> [_ w381]
                  tunnel: w344 -> [_ w378]
                  tunnel: w349 -> [_ w377]
                  frame False {
                  }
                  frame True {
                    n132 = Index Array(array=w381, index #1=0 ("index"), index #2=1 ("index")) -> (element #1=w370:string, element #2=w375:string)
                    n133 = Format Into String(format string="Warning\n%s=%.0f %s=%.0f", w370, w378, w375, w377) -> (resulting string=w373:string)  [unwired: 2 in, 1 out]
                    n134 = call "Fast_string_Replace.vi"("Replace match with:"=" ", "Input String"=w370, "matchThis"=":" ("regular expression")) -> ("Output String"=w369:string)  [unwired: 1 in, 1 out]
                    n135 = call "Server_Emails.vi"("Client Name Contains"="EnFlo_Tunnel", "Message"=w373, "Subject"=w369) -> ()  [unwired: 2 in, 3 out]
                  }
                }
                n136 = case shown="True" w335 {
                  tunnel: w348 -> [_ _]
                  tunnel: w347 -> [_ w368]
                  tunnel: w339 -> [_ w365]
                  tunnel: w346 -> [_ w364]
                  frame False {
                  }
                  frame True {
                    n137 = Index Array(array=w368, index #1=2 ("index"), index #2=3 ("index")) -> (element #1=w359:string, element #2=w362:string)
                    n138 = Format Into String(format string="Warning\n%s=%.0f %s=%.0f", w359, w365, w362, w364) -> (resulting string=w360:string)  [unwired: 2 in, 1 out]
                    n139 = call "Fast_string_Replace.vi"("Replace match with:"=" ", "Input String"=w359, "matchThis"=":" ("regular expression")) -> ("Output String"=w358:string)  [unwired: 1 in, 1 out]
                    n140 = call "Server_Emails.vi"("Client Name Contains"="EnFlo_Tunnel", "Message"=w360, "Subject"=w358) -> ()  [unwired: 2 in, 3 out]
                  }
                }
              }
            }
          }
          frame #7 {
            n141 = case shown="True" w384 {
              tunnel: w382 -> [_ w389]
              tunnel: ["" w390] -> w383
              tunnel: w382 -> [_ w387]
              tunnel: w382 -> [_ w386]
              frame False {
              }
              frame True {
                w391 = string[] ["EnFlo_Tunnel:Temp:Pre_Inlet_Y=1500_Z=450", "EnFlo_Tunnel:Temp:Pre_Inlet_Y=-1500_Z=450", "EnFlo_Tunnel:Temp:Pre_Inlet_Y=1000_Z=450", "EnFlo_Tunnel:Temp:Pre_Inlet_Y=-1000_Z=450", "EnFlo_Tunnel:Temp:Pre_Inlet_Y=500_Z=450"] ("Sub set")
                n142 = Subtract(x=w389, y=300.0 ("x-y")) -> (x-y=w403:dbl)
                n143 = call "Get_ADAM_averages_client.vi"("No of averages"=1, "End time"=w389, "Start time"=w403, "ADAM Ch Names"=w391) -> ("Messages"=w390:string, "DBL values"=w407:dbl[][])  [unwired: 3 in, 3 out]
                n144 = Index Array(array=w407, index (row)=1 ("disabled index (col)")) -> (element=w402:dbl[])  [unwired: 1 in]
                n145 = Array Subset(array=w402, index=1, length=5) -> (w400:dbl[])
                n146 = Array Max & Min(array=w400) -> (max value=w397:dbl, max index (indices)=w395:i32, min value=w399:dbl, min index (indices)=w396:i32)
                n147 = Subtract(x=w397, y=w399) -> (x-y=w392:dbl)
                n148 = Index Array(array=w391, index=w396) -> (element=w393:string)
                n149 = Greater Or Equal?(x=w392, y=0.3) -> (x >= y?=w388:bool)
                n150 = Index Array(array=w391, index=w395) -> (element=w394:string)
                n151 = case shown="True" w388 {
                  tunnel: w394 -> [_ w423]
                  tunnel: w393 -> [_ w422]
                  tunnel: w392 -> [_ w421]
                  tunnel: w387 -> [_ w413]
                  tunnel: w386 -> [_ w411]
                  frame False {
                  }
                  frame True {
                    n152 = Subtract(x=w413, y=1200.0) -> (x-y=w416:dbl)
                    n153 = call "Get_ADAM_averages_client.vi"("No of averages"=20, "End time"=w411, "Start time"=w416, "ADAM Ch Names"=string[] ["EnFlo_Tunnel:Reference:Velocity"]) -> ("DBL values"=w419:dbl[][])  [unwired: 3 in, 4 out]
                    n154 = global read "EnFlo_Tunnel_Global.vi" "Minimum Ref Velocity for taking Results"() -> (w417:dbl)
                    n155 = Index Array(array=w419, index (col)=1 ("disabled index (col)")) -> (element=w418:dbl[])  [unwired: 1 in]
                    n156 = Greater Or Equal?(x=w418, y=w417) -> (x >= y?=w420:bool[])
                    n157 = And Array Elements(Boolean array=w420) -> (logical AND=w409:bool)
                    n158 = case shown="True" w409 {
                      tunnel: w421 -> [_ w426]
                      tunnel: w422 -> [_ w425]
                      tunnel: w423 -> [_ w424]
                      frame False {
                      }
                      frame True {
                        n159 = Format Into String(format string="The %s is %.2f degC more than %s.\\n Check the inlet fans are operating correctly." ("Format String"), w424, w426, w425) -> (resulting string=w428:string)  [unwired: 2 in, 1 out]
                        n160 = call "Server_Emails.vi"("Client Name Contains"="EnFlo_Tunnel", "Message"=w428, "Subject"="Large Inlet Temperature Variation" ("Error Type")) -> ()  [unwired: 2 in, 3 out]
                      }
                    }
                  }
                }
              }
            }
          }
          frame #8 {
            w440 = "EnFlo_Tunnel:Motor:Enable"
            w443 = "A_Tunnel:Motor:Enable"
            w452 = "Aero_Tunnel:Motor:Enable"
            # "Turning off Tunnel Drives if not used for more than"
            n161 = Build Array("A_Tunnel:Speed:Dem Velocity", w443) -> (w450:string[])
            n162 = Build Array("EnFlo_Tunnel:Speed:Dem Velocity", w440) -> (w431:string[])
            n163 = Build Array (concatenate)("Aero_Tunnel:Speed:Dem Velocity", w452, w450, w431) -> (w458:string[])
            n164 = call "Get_Channel_averages.vi"("Desired Ch Names"=w458, "Averaging time (mins)"=20.0) -> ("number"=w432:dbl[])  [unwired: 1 in, 2 out]
            n165 = Index Array(array=w432, index #1=2 ("index"), index #2=3 ("index")) -> (element #1=w445:dbl, element #2=w444:dbl)
            n166 = Index Array(array=w432, index #1=4 ("index"), index #2=5 ("index")) -> (element #1=w438:dbl, element #2=w439:dbl)
            n167 = Index Array(array=w432) -> (element #1=w457:dbl, element #2=w456:dbl)  [unwired: 2 in]
            n168 = Equal To 0?(x=w445) -> (x = 0?=w447:bool)
            n169 = Greater Than 0?(x=w444) -> (x > 0?=w446:bool)
            n170 = Equal To 0?(x=w438) -> (x = 0?=w436:bool)
            n171 = Greater Than 0?(x=w439) -> (x > 0?=w437:bool)
            n172 = Equal To 0?(x=w457) -> (x = 0?=w454:bool)
            n173 = Greater Than 0?(x=w456) -> (x > 0?=w455:bool)
            n174 = And(x=w447, y=w446) -> (x .and. y?=w442:bool)
            n175 = case shown="True" w442 {
              tunnel: w443 -> [_ w471]
              frame False {
              }
              frame True {
                n176 = Build Array(w471) -> (w470:string[])
                n177 = Build Array(0.0) -> (w469:dbl[])
                n178 = call "ASYNC_Adam_server.vi"("Values"=w469, "Channel Names"=w470) -> ()  [unwired: 1 in, 3 out]
              }
            }
            n179 = And(x=w436, y=w437) -> (x .and. y?=w441:bool)
            n180 = case shown="True" w441 {
              tunnel: w440 -> [_ w467]
              frame False {
              }
              frame True {
                n181 = Build Array(w467) -> (w466:string[])
                n182 = Build Array(0.0) -> (w465:dbl[])
                n183 = call "ASYNC_Adam_server.vi"("Values"=w465, "Channel Names"=w466) -> ()  [unwired: 1 in, 3 out]
                n184 = call "Ch_Active_Control.vi"("Match"="EnFlo_Tunnel:Drive:In Standby", "Activate Channels?"=FALSE, "Control on"=Channel_State_Control."Channel Name") -> ()  [unwired: 1 in, 2 out]
              }
            }
            n185 = And(x=w454, y=w455) -> (x .and. y?=w453:bool)
            n186 = case shown="True" w453 {
              tunnel: w452 -> [_ w475]
              frame False {
              }
              frame True {
                n187 = Build Array(w475) -> (w474:string[])
                n188 = Build Array(0.0) -> (w473:dbl[])
                n189 = call "ASYNC_Adam_server.vi"("Values"=w473, "Channel Names"=w474) -> ()  [unwired: 1 in, 3 out]
              }
            }
          }
          frame #9 {
            # "Code to only execute \"Zero Uref Pressure Transducers\" every 9 minutes"
            n190 = while {
              shift-right: [w486] -> _
              shift-left: _ -> [w484]
              tunnel: [w485] -> w476
              stop <- TRUE stop-if-true
              n191 = Less?(x=w484, y=2) -> (x < y?=w487:bool)
              n192 = case shown="False" w487 {
                tunnel: [0 w493] -> w486
                tunnel: ["Zero Uref Pressure Transducers" "EnFlo Tunnel Checks"] -> w485
                tunnel: w484 -> [_ w494]
                frame False {
                }
                frame True {
                  n193 = Add(x=w494, y=1) -> (x+y=w493:i32)
                }
              }
            }
            n194 = Concatenate Strings(w483, w477, w482, w480, w479, w478) -> (w481:string)
          }
        }
      }
      frame "Zero Uref Pressure Transducers" {
        w502 = string[] ["A_Tunnel:Speed:Pitot (Pa)", "Aero_Tunnel:Speed:Pitot (Pa)", "D_Tunnel:Speed:Pitot (Pa)", "A_Tunnel:Contraction:Delta P"]  # Channel to Zero
        w503 = string[] ["A_Tunnel:Motor:Enable", "Aero_Tunnel:Motor:Enable", "D_Tunnel:Motor:Enable", "A_Tunnel:Motor:Enable"]  # Is tunnel Running?
        # "These two channel name arrays need to be editted at the same time"
        # "This frame only Executes every 9 minutes"
        n195 = Build Array (concatenate)(w503, w502) -> (w507:string[])
        n196 = Array Size(array=w502) -> (size(s)=w506:i32)
        n197 = call "Get_Channel_averages.vi"("Desired Ch Names"=w507, "Averaging time (mins)"=7.0) -> ("number"=w505:dbl[])  [unwired: 1 in, 2 out]
        n198 = Split 1D Array(array=w505, index=w506) -> (first subarray=w504:dbl[], second subarray=w499:dbl[])
        n199 = for {
          tunnel: w504 -> [w524] mode=indexing
          tunnel: [w523] -> w500 mode=indexing if=w521
          tunnel: w502 -> [w523] mode=indexing
          tunnel: [w522] -> w498 mode=indexing if=w521
          tunnel: w499 -> [w522] mode=indexing
          n200 = Equal To 0?(x=w524) -> (x = 0?=w521:bool)
        }
        n201 = Empty Array?(array=w500) -> (empty?=w501:bool)
        n202 = case shown="False" w501 {
          tunnel: w500 -> [w514 _]
          tunnel: w498 -> [w512 _]
          frame False {
            n203 = call "Get_Current_Scan_server.vi"("Desired Channels"=w514) -> ("Ch Description Array"=w513:T6[])  [unwired: 2 out]
            n204 = for {
              tunnel: w513 -> [w516] mode=indexing
              tunnel: w512 -> [w517] mode=indexing
              tunnel: [w515] -> w511 mode=indexing
              n205 = in-place {
                in-place-border: w517 -> [w520]
                n206 = in-place-cluster #3(w516) -> ("A"=w519:dbl)
                n207 = Subtract(x=w519, y=w520) -> (x-y=w518:dbl)
                n208 = in-place-cluster #3("A"=w518) -> (w515:T6)
              }
            }
            n209 = call "Update_Ch_Discription_server.vi"("Mode"=T3."Append to Global", "Channels to update In"=w511) -> ()  [unwired: 1 in, 1 out]
          }
          frame True {
          }
        }
      }
      frame "EnFlo Tunnel Checks" {
        n210 = stacked-sequence {
          seq-local: [w538 _ _ _ _ _] -> [_ w569 _ _ _ _]
          seq-local: [_ w568 _ _ _ _] -> [_ _ _ _ _ w719]
          seq-local: [w535 _ _ _ _ _] -> [_ _ _ _ _ w720]
          seq-local: [_ _ w595 _ _ _] -> [_ _ _ w613 _ _]
          seq-local: [_ _ _ _ w678 _] -> [_ _ _ _ _ w717]
          seq-local: [w534 _ _ _ _ _] -> [_ _ _ w607 _ _]
          tunnel: w531 -> [w541 w571 w605 w612 w680 _]
          tunnel: w530 -> [w540 w570 w604 w611 w679 _]
          tunnel: [w542 _ _ _ _ _] -> w529
          tunnel: w528 -> [_ _ _ w610 _ _]
          tunnel: w527 -> [_ _ _ w609 _ _]
          tunnel: w526 -> [_ _ _ _ _ w721]
          tunnel: [_ _ _ _ _ w718] -> w525
          frame #0 {
            n211 = call "Read_value_of_earlier_Ch.vi"("Desired Ch to Read"="EnFlo_Tunnel:Minimum Uref:Happy", "Ch names"=w540, "Present scan array"=w541) -> ("Value"=w544:dbl, "Scan comment"=w536:string)  [unwired: 1 in]
            n212 = Greater?(x=w544, y=0.5) -> (0:w534:bool)
            n213 = case shown="True" w534 {
              tunnel: [w547 w560] -> w542
              tunnel: w541 -> [_ w558]
              tunnel: w540 -> [_ w557]
              tunnel: "Check EnFlo tweak factor?" -> [w547 w559]
              tunnel: [FALSE w551] -> w538
              tunnel: ["" w548] -> w537
              frame False {
              }
              frame True {
                n214 = call "Read_value_of_earlier_Ch.vi"("Desired Ch to Read"="EnFlo_Tunnel:Bus Bar + Heaters:Enable", "Ch names"=w557, "Present scan array"=w558) -> ("Value"=w555:dbl, "Scan comment"=w550:string)  [unwired: 1 in]
                n215 = call "Read_value_of_earlier_Ch.vi"("Desired Ch to Read"="EnFlo_Tunnel:Enable:Inlet_Lamps", "Ch names"=w557, "Present scan array"=w558) -> ("Value"=w554:dbl, "Scan comment"=w549:string)  [unwired: 1 in]
                n216 = Build Array(w555, w554) -> (w553:dbl[])
                n217 = Greater?(x=w553, y=0.5) -> (0:w552:bool[])
                n218 = And Array Elements(Boolean array=w552) -> (logical AND=w551:bool)
                n219 = case shown="True" w551 {
                  tunnel: [w563 w564] -> w560
                  tunnel: w559 -> [w563 w567]
                  frame False {
                  }
                  frame True {
                    n220 = Select(t=w567, s="Manual Control of Lamps", f="Lamp control") -> (s? t:f=w564:string)
                  }
                }
                n221 = Concatenate Strings(w550, w549) -> (w548:string)
              }
            }
            n222 = Concatenate Strings(w537, w536) -> (w535:string)
          }
          frame #1 {
            n223 = case shown="False" w569 {
              tunnel: w571 -> [w576 _]
              tunnel: w570 -> [w575 _]
              tunnel: [w572 ""] -> w568
              frame False {
                n224 = for {
                  tunnel: [w582] -> w579 mode=indexing if=w583
                  tunnel: [0.0 ("Value")] -> w578 mode=indexing if=w583
                  tunnel: string[] ["EnFlo_Tunnel:Inlet_Lamp Y=-1313_Z=1125:Dem_Power(%)", "EnFlo_Tunnel:Inlet_Lamp Y=-1313_Z=375:Dem_Power(%)", "EnFlo_Tunnel:Inlet_Lamp Y=-438_Z=1125:Dem_Power(%)", "EnFlo_Tunnel:Inlet_Lamp Y=-438_Z=375:Dem_Power(%)", "EnFlo_Tunnel:Inlet_Lamp Y=438_Z=1125:Dem_Power(%)", "EnFlo_Tunnel:Inlet_Lamp Y=438_Z=375:Dem_Power(%)", "EnFlo_Tunnel:Inlet_Lamp Y=1313_Z=1125:Dem_Power(%)", "EnFlo_Tunnel:Inlet_Lamp Y=1313_Z=375:Dem_Power(%)"] ("Sub set") -> [w582] mode=indexing
                  tunnel: w576 -> [w586]
                  tunnel: w575 -> [w585]
                  tunnel: [w580] -> w574 mode=indexing
                  n225 = call "Read_value_of_earlier_Ch.vi"("Desired Ch to Read"=w582, "Ch names"=w585, "Present scan array"=w586) -> ("Value"=w584:dbl, "Scan comment"=w580:string)  [unwired: 1 in]
                  n226 = Not Equal To 0?(x=w584) -> (x != 0?=w583:bool)
                }
                n227 = call "ASYNC_Adam_server.vi"("Values"=w578, "Channel Names"=w579) -> ("Scan Comments"=w573:string[])  [unwired: 1 in, 2 out]
                n228 = Concatenate Strings(w574, w573) -> (w572:string)
              }
              frame True {
              }
            }
          }
          frame #2 {
            n229 = call "Read_Earlier_Channels.vi"("Present scan array"=w605, "Ch names"=w604, "Desired Channels"=string[] ["EnFlo_Tunnel:Bus Bar + Heaters:Enable", "EnFlo_Tunnel:Speed:Dem Velocity", "EnFlo_Tunnel:Reference:Velocity", "EnFlo_Tunnel:Shutting:Down"]) -> ("Index 0"=w602:dbl, "Index 1"=w598:dbl, "Index 2"=w597:dbl, "Index 3"=w590:dbl)  [unwired: 2 out]
            n230 = Less?(x=w590, y=0.5) -> (x < y?=w588:bool)
            n231 = Greater?(x=w602, y=0.5) -> (0:w596:bool)
            n232 = call "In_Range_check.vi"("±"=0.25, "%"=30.0, "Mode"=In_Range."% & ±", "Value"=w597, "Setpoint"=w598) -> ("In Range"=w592:bool)  [unwired: 2 in]
            n233 = feedback #4() -> (w594:dbl[])  [unwired: 1 in]
            n234 = call "On_Off_with_hysteresis.vi"("Shift In"=w594, "New Value"=w592) -> ("Shift Out"=w593:dbl[], "Output State"=w591:bool)  [unwired: 4 in]
            n235 = feedback-in #4(w593) -> ()
            n236 = Compound Arithmetic op=AND(w596, w591, w588) -> (w595:bool)
          }
          frame #3 {
            n237 = case shown="True" w613 {
              tunnel: w610 -> [_ w629]
              tunnel: w612 -> [w617 w628]
              tunnel: w611 -> [w616 w627]
              tunnel: w609 -> [_ w626]
              tunnel: "EnFlo_Tunnel:Power:Inlet_Door_Heaters" ("Desired Ch to Read") -> [w615 w625]
              tunnel: w607 -> [_ w624]
              frame False {
                n238 = call "Read_value_of_earlier_Ch.vi"("Desired Ch to Read"=w615, "Ch names"=w616, "Present scan array"=w617) -> ("Value"=w619:dbl)  [unwired: 1 in, 1 out]
                n239 = Greater?(x=w619, y=0.5) -> (0:w614:bool)
                n240 = case shown="False" w614 {
                  tunnel: w615 -> [_ w621]
                  frame False {
                  }
                  frame True {
                    n241 = Build Array(w621) -> (w623:string[])
                    n242 = Build Array(0.0 ("element")) -> (w622:dbl[])
                    n243 = call "ASYNC_Adam_server.vi"("Values"=w622, "Channel Names"=w623) -> ()  [unwired: 1 in, 3 out]
                  }
                }
              }
              frame True {
                n244 = stacked-sequence {
                  seq-local: [w634 _] -> [_ w654]
                  seq-local: [w633 _] -> [_ w652]
                  tunnel: w629 -> [w649 _]
                  tunnel: w628 -> [_ w657]
                  tunnel: w627 -> [_ w656]
                  tunnel: w626 -> [w630 _]
                  tunnel: w625 -> [_ w655]
                  tunnel: w624 -> [_ w653]
                  frame #0 {
                    w637 = 2.0 ("y")
                    # "Delta T"
                    n245 = Subtract(x=w649, y=w630) -> (x-y=w648:dbl)
                    n246 = call "Get_ADAM_averages_server.vi"("No of averages"=1, "End time"=w649, "Start time"=w648, "Clients time"=w649, "ADAM Ch Names"=string[] ["EnFlo_Tunnel:Temp:Pre_Inlet_Y=-1500_Z=450", "EnFlo_Tunnel:Temp:Pre_Inlet_Y=-1000_Z=450", "EnFlo_Tunnel:Temp:Pre_Inlet_Y=1500_Z=450", "EnFlo_Tunnel:Temp:Pre_Inlet_Y=1000_Z=450"]) -> ("DBL values"=w646:dbl[][])  [unwired: 1 in, 4 out]
                    n247 = Index Array(array=w646, index (row)=0) -> (element=w644:dbl[])  [unwired: 1 in]
                    n248 = Index Array(array=w644) -> (element #2=w642:dbl, element #3=w643:dbl, element #4=w641:dbl, element #5=w640:dbl)  [unwired: 5 in, 1 out]
                    n249 = Add(x=w642, y=w643) -> (x+y=w639:dbl)
                    n250 = Add(x=w641, y=w640) -> (x+y=w638:dbl)
                    n251 = Divide(x=w639, y=w637) -> (x/y=w631:dbl)
                    n252 = Divide(x=w638, y=w637) -> (x/y=w632:dbl)
                    n253 = Subtract(x=w631, y=w632) -> (x-y=w634:dbl)
                    n254 = Absolute Value(x=w634) -> (abs(x)=w636:dbl)
                    n255 = Greater?(x=w636, y="Deadband Delta T") -> (0:w633:bool)
                  }
                  frame #1 {
                    n256 = And(x=w653, y=w652) -> (x .and. y?=w651:bool)
                    n257 = case shown="True" w651 {
                      tunnel: w657 -> [_ w676]
                      tunnel: w656 -> [_ w675]
                      tunnel: w654 -> [_ w674]
                      tunnel: w655 -> [_ w659]
                      frame False {
                      }
                      frame True {
                        n258 = Multiply(x=w674, y="Kp") -> (x*y=w672:dbl)
                        n259 = In Range and Coerce(upper limit=1.0, x=w672, lower limit=-1.0) -> (coerced(x)=w668:dbl)  [unwired: 1 out]
                        n260 = call "Read_value_of_earlier_Ch.vi"("Desired Ch to Read"=w659, "Ch names"=w675, "Present scan array"=w676) -> ("Value"=w669:dbl)  [unwired: 1 in, 1 out]
                        n261 = Add(x=w669, y=w668) -> (x+y=w665:dbl)
                        n262 = In Range and Coerce(upper limit=100.0, x=w665, lower limit=0.0) -> (coerced(x)=w661:dbl)  [unwired: 1 out]
                        n263 = Not A Number/Path/Refnum?(number/path/refnum=w661) -> (NaN/Path/Refnum?=w662:bool)
                        n264 = Select(t=0.0, s=w662, f=w661) -> (s? t:f=w658:dbl)
                        n265 = Build Array(w659) -> (w664:string[])
                        n266 = Build Array(w658) -> (w663:dbl[])
                        n267 = call "ASYNC_Adam_server.vi"("Values"=w663, "Channel Names"=w664) -> ()  [unwired: 1 in, 3 out]
                      }
                    }
                  }
                }
              }
            }
          }
          frame #4 {
            n268 = global read "EnFlo_Tunnel_Global.vi" "Minimum Ref Velocity"() -> (w693:dbl)
            n269 = Build Array("EnFlo_Tunnel:Speed:Dem Velocity" ("Desired Ch to Read")) -> (w691:string[])
            n270 = call "Read_Earlier_Channels.vi"("Present scan array"=w680, "Ch names"=w679, "Desired Channels"=w691) -> ("Scan comments"=w682:string, "Index 0"=w692:dbl)  [unwired: 4 out]
            n271 = Greater?(x=w692, y=w693) -> (0:w689:bool)
            n272 = Boolean To (0,1)(Boolean=w689) -> (0, 1=w686:i16)
            n273 = feedback #5() -> (w687:dbl[])  [unwired: 1 in]
            n274 = call "Running_Ch_Average.vi"("Shift In"=w687, "History length"=15, "Reset Average after Seconds"=120.0, "New Value"=w686) -> ("Shift Out"=w688:dbl[], "mean"=w683:dbl)  [unwired: 1 in, 1 out]
            n275 = feedback-in #5(w688) -> ()
            n276 = Equal To 0?(x=w683) -> (x = 0?=w684:bool)
            n277 = case shown="True" w684 {
              tunnel: [w694 w705] -> w678
              tunnel: w682 -> [w694 w704]
              tunnel: w679 -> [_ w703]
              tunnel: w680 -> [_ w702]
              tunnel: "EnFlo_Tunnel:Heater:Enable" -> [_ w695]
              frame False {
              }
              frame True {
                w698 = "EnFlo_Tunnel:Bus Bar + Heaters:Enable"
                n278 = call "Read_value_of_earlier_Ch.vi"("Desired Ch to Read"=w698, "Ch names"=w703, "Present scan array"=w702) -> ("Value"=w701:dbl)  [unwired: 1 in, 1 out]
                n279 = Initialize Array("", 0 ("dimension size")) -> (w699:string[])
                n280 = Greater Than 0?(x=w701) -> (x > 0?=w700:bool)
                n281 = case shown="True" w700 {
                  tunnel: w698 -> [_ w714]
                  tunnel: w699 -> [w711 w713]
                  tunnel: [w711 w712] -> w697
                  frame False {
                  }
                  frame True {
                    n282 = Build Array (concatenate)(w714, w713) -> (w712:string[])
                  }
                }
                n283 = Build Array (concatenate)(w697, w695) -> (w696:string[])
                n284 = for {
                  tunnel: [w716] -> w708 mode=indexing
                  tunnel: w696 -> [w716] mode=indexing
                  tunnel: [0.0] -> w707 mode=indexing
                }
                n285 = call "ASYNC_Adam_server.vi"("Values"=w707, "Channel Names"=w708) -> ("Scan Comments"=w706:string[])  [unwired: 1 in, 2 out]
                n286 = Concatenate Strings(w704, w706) -> (w705:string)
              }
            }
          }
          frame #5 {
            n287 = Concatenate Strings(w717, w721, w720, w719) -> (w718:string)
          }
        }
      }
      frame "Lamp control" {
        # "Heaters\nOn"
        # "Inlet"
        n288 = stacked-sequence {
          seq-local: [_ _ w759 _ _ _ _] -> [_ _ _ _ _ w848 w922]
          seq-local: [_ _ w757 _ _ _ _] -> [_ _ _ w811 w821 w847 _]
          seq-local: [_ _ _ w808 _ _ _] -> [_ _ _ _ w819 w846 _]
          seq-local: [_ _ _ _ _ w839 _] -> [_ _ _ _ _ _ w911]
          seq-local: [_ w750 _ _ _ _ _] -> [_ _ _ _ _ w845 w905]
          seq-local: [w732 _ _ _ _ _ _] -> [_ _ _ _ w822 w834 _]
          seq-local: [w731 _ _ _ _ _ _] -> [_ _ w755 _ w820 _ _]
          seq-local: [_ _ _ _ w818 _ _] -> [_ _ _ _ _ w833 _]
          seq-local: [w730 _ _ _ _ _ _] -> [_ _ _ _ _ _ w893]
          tunnel: w728 -> [_ _ _ w813 _ _ _]
          tunnel: w727 -> [_ _ _ w812 _ _ _]
          tunnel: w726 -> [w736 _ _ _ _ _ w921]
          tunnel: w725 -> [w735 _ _ _ _ _ w920]
          tunnel: [_ _ _ _ _ _ "Check EnFlo tweak factor?"] -> w724
          tunnel: w723 -> [_ _ _ _ _ _ w894]
          tunnel: [_ _ _ _ _ _ w890] -> w722
          frame #0 {
            n289 = call "Heater_Enable_Chs.vi"() -> ("Inlet Heaters"=w738:T12)  [unwired: 4 in, 5 out]
            n290 = Unbundle By Name(w738) -> ("Connected Items"=w737:string[])
            n291 = for {
              tunnel: w737 -> [w745] mode=indexing
              tunnel: w736 -> [w744]
              tunnel: w735 -> [w743]
              tunnel: [w742] -> w734 mode=indexing
              tunnel: [w741] -> w730 mode=indexing
              n292 = call "Read_value_of_earlier_Ch.vi"("Desired Ch to Read"=w745, "Ch names"=w743, "Present scan array"=w744) -> ("Value"=w742:dbl, "Scan comment"=w741:string)  [unwired: 1 in]
            }
            n293 = Add Array Elements(numeric array=w734) -> (sum=w733:dbl)
            n294 = Greater Than 0?(x=w733) -> (x > 0?=w732:bool)
            n295 = case shown="True" w732 {
              tunnel: [string[] [] ("Sub set") string[] ["EnFlo_Tunnel:Temp:Inlet_Y=0_Z=50", "EnFlo_Tunnel:Temp:Inlet_Y=0_Z=150", "EnFlo_Tunnel:Temp:Inlet_Y=0_Z=250", "EnFlo_Tunnel:Temp:Inlet_Y=0_Z=350", "EnFlo_Tunnel:Temp:Inlet_Y=0_Z=450", "EnFlo_Tunnel:Temp:Inlet_Y=0_Z=550", "EnFlo_Tunnel:Temp:Inlet_Y=0_Z=650", "EnFlo_Tunnel:Temp:Inlet_Y=0_Z=750", "EnFlo_Tunnel:Temp:Inlet_Y=0_Z=850", "EnFlo_Tunnel:Temp:Inlet_Y=0_Z=950", "EnFlo_Tunnel:Temp:Inlet_Y=0_Z=1050", "EnFlo_Tunnel:Temp:Inlet_Y=0_Z=1150", "EnFlo_Tunnel:Temp:Inlet_Y=0_Z=1250", "EnFlo_Tunnel:Temp:Inlet_Y=0_Z=1350", "EnFlo_Tunnel:Temp:Inlet_Y=0_Z=1450"] ("Sub set")] -> w731
              frame False {
              }
              frame True {
              }
            }
          }
          frame #1 {
            w747 = 750.0 ("Y Scale.Offset and Multiplier:Multiplier")
            w746 = 0.0 ("Y Scale.Offset and Multiplier:Offset")
            w749 = 875.0 ("X Scale.Offset and Multiplier:Multiplier")
            w748 = -1750.0 ("X Scale.Offset and Multiplier:Offset")
            n296 = Initialize Array(0.0, 2 ("dimension size"), 4 ("dimension size")) -> (w750:dbl[][])
            n297 = property on="Temperature" class="IntGraph (strict)"("XScale.Multiplier"=w749, "XScale.Offset"=w748, "YScale.Multiplier"=w747, "YScale.Offset"=w746) -> ()  [unwired: 2 in, 2 out]
            n298 = property on="Power" class="IntGraph (strict)"("XScale.Multiplier"=w749, "XScale.Offset"=w748, "YScale.Multiplier"=w747, "YScale.Offset"=w746) -> ()  [unwired: 2 in, 2 out]
          }
          frame #2 {
            n299 = for {
              N: 8 -> [_]
              tunnel: [w766] -> w759 mode=indexing
              tunnel: [w762] -> w756 mode=concatenating
              i -> [w765]
              n300 = Increment(x=w765) -> (x+1=w764:i32)
              n301 = case shown="7" w764 {
                tunnel: [string[] ["EnFlo_Tunnel:Temp:Inlet_Y=-1500_Z=950", "EnFlo_Tunnel:Temp:Inlet_Y=-1000_Z=950", "EnFlo_Tunnel:Temp:Inlet_Y=-1500_Z=1450", "EnFlo_Tunnel:Temp:Inlet_Y=-1000_Z=1450"] ("subarray") string[] ["EnFlo_Tunnel:Temp:Inlet_Y=-1500_Z=50", "EnFlo_Tunnel:Temp:Inlet_Y=-1000_Z=50", "EnFlo_Tunnel:Temp:Inlet_Y=-1500_Z=450", "EnFlo_Tunnel:Temp:Inlet_Y=-1000_Z=450"] ("subarray") string[] ["EnFlo_Tunnel:Temp:Inlet_Y=-500_Z=950", "EnFlo_Tunnel:Temp:Inlet_Y=0_Z=950", "EnFlo_Tunnel:Temp:Inlet_Y=-500_Z=1450", "EnFlo_Tunnel:Temp:Inlet_Y=0_Z=1450"] ("subarray") string[] ["EnFlo_Tunnel:Temp:Inlet_Y=-500_Z=50", "EnFlo_Tunnel:Temp:Inlet_Y=0_Z=50", "EnFlo_Tunnel:Temp:Inlet_Y=-500_Z=450", "EnFlo_Tunnel:Temp:Inlet_Y=0_Z=450"] ("subarray") string[] ["EnFlo_Tunnel:Temp:Inlet_Y=500_Z=950", "EnFlo_Tunnel:Temp:Inlet_Y=0_Z=950", "EnFlo_Tunnel:Temp:Inlet_Y=500_Z=1450", "EnFlo_Tunnel:Temp:Inlet_Y=0_Z=1450"] ("subarray") string[] ["EnFlo_Tunnel:Temp:Inlet_Y=500_Z=50", "EnFlo_Tunnel:Temp:Inlet_Y=0_Z=50", "EnFlo_Tunnel:Temp:Inlet_Y=500_Z=450", "EnFlo_Tunnel:Temp:Inlet_Y=0_Z=450"] ("subarray") string[] ["EnFlo_Tunnel:Temp:Inlet_Y=1500_Z=950", "EnFlo_Tunnel:Temp:Inlet_Y=1000_Z=950", "EnFlo_Tunnel:Temp:Inlet_Y=1500_Z=1450", "EnFlo_Tunnel:Temp:Inlet_Y=1000_Z=1450"] ("subarray") string[] ["EnFlo_Tunnel:Temp:Inlet_Y=1500_Z=50", "EnFlo_Tunnel:Temp:Inlet_Y=1000_Z=50", "EnFlo_Tunnel:Temp:Inlet_Y=1500_Z=450", "EnFlo_Tunnel:Temp:Inlet_Y=1000_Z=450"] ("subarray")] -> w762
                tunnel: [dbl[] [1.0, 1.0, 1.0, 1.0] ("subarray") dbl[] [1.0, 1.0, 1.0, 1.0] ("subarray") dbl[] [1.0, 0.5, 1.0, 0.5] ("subarray") dbl[] [1.0, 0.5, 1.0, 0.5] ("subarray") dbl[] [1.0, 0.5, 1.0, 0.5] ("subarray") dbl[] [1.0, 0.5, 1.0, 0.5] ("subarray") dbl[] [1.0, 1.0, 1.0, 1.0] ("subarray") dbl[] [1.0, 1.0, 1.0, 1.0] ("subarray")] -> w767
                tunnel: ["EnFlo_Tunnel:Inlet_Lamp Y=-1313_Z=1125:Dem_Power(%)" ("Ch Name") "EnFlo_Tunnel:Inlet_Lamp Y=-1313_Z=375:Dem_Power(%)" ("Ch Name") "EnFlo_Tunnel:Inlet_Lamp Y=-438_Z=1125:Dem_Power(%)" ("Ch Name") "EnFlo_Tunnel:Inlet_Lamp Y=-438_Z=375:Dem_Power(%)" ("Ch Name") "EnFlo_Tunnel:Inlet_Lamp Y=438_Z=1125:Dem_Power(%)" ("Ch Name") "EnFlo_Tunnel:Inlet_Lamp Y=438_Z=375:Dem_Power(%)" ("Ch Name") "EnFlo_Tunnel:Inlet_Lamp Y=1313_Z=1125:Dem_Power(%)" ("Ch Name") "EnFlo_Tunnel:Inlet_Lamp Y=1313_Z=375:Dem_Power(%)" ("Ch Name")] -> w763
                tunnel: [1 0 1 0 1 0 1 0] -> w761
                tunnel: [0 0 1 1 2 2 3 3] -> w760
                frame 1, Default {
                }
                frame 2 {
                }
                frame 3 {
                }
                frame 4 {
                }
                frame 5 {
                }
                frame 6 {
                }
                frame 7 {
                }
                frame 8 {
                }
              }
              n302 = Bundle("Ch Name"=w763, "subarray"=w762, "subarray"=w767, w761, w760) -> (w766:T13)  [unwired: 1 in]
            }
            n303 = Build Array (concatenate)(w755, w756) -> (w754:string[])
            n304 = call "Analyse_string_array.vi"("String array"=w754) -> ("Unique strings"=w757:string[])  [unwired: 1 in, 1 out]
          }
          frame #3 {
            # "Averaging time seconds"
            n305 = Subtract(x=w813, y=w812) -> (x-y=w817:dbl)
            n306 = call "Get_ADAM_averages_server.vi"("No of averages"=1, "End time"=w813, "Start time"=w817, "Clients time"=w813, "ADAM Ch Names"=w811) -> ("DBL values"=w815:dbl[][])  [unwired: 1 in, 4 out]
            n307 = Index Array(array=w815, index (row)=0) -> (element=w810:dbl[])  [unwired: 1 in]
            n308 = Array Subset(array=w810, index=1) -> (w808:dbl[])  [unwired: 1 in]
          }
          frame #4 {
            n309 = case shown="True" w822 {
              tunnel: w821 -> [_ w827]
              tunnel: w820 -> [_ w826]
              tunnel: w819 -> [_ w825]
              tunnel: [dbl[] [] w824] -> w818
              frame False {
              }
              frame True {
                n310 = for {
                  tunnel: w827 -> [w831]
                  tunnel: w826 -> [w830] mode=indexing
                  tunnel: w825 -> [w829]
                  tunnel: [w828] -> w824 mode=indexing
                  n311 = Search 1D Array(1D array=w831, element=w830) -> (index of element=w832:i32)  [unwired: 1 in]
                  n312 = Index Array(array=w829, index=w832) -> (element=w828:dbl)
                }
              }
            }
          }
          frame #5 {
            n313 = for {
              tunnel: w848 -> [w863] mode=indexing
              tunnel: w847 -> [w862]
              tunnel: w846 -> [w860]
              tunnel: [w851] -> w839 mode=indexing
              shift-right: [w854] -> w844
              shift-left: w845 -> [w855]
              tunnel: w834 -> [w850]
              tunnel: w833 -> [w849]
              n314 = Unbundle(w863) -> ("subarray"=w861:string[], "subarray"=w859:dbl[], w853:i32, w852:i32)  [unwired: 1 out]
              n315 = for {
                tunnel: w862 -> [w873]
                tunnel: w861 -> [w865] mode=indexing
                tunnel: w860 -> [w872]
                tunnel: w859 -> [w870] mode=indexing
                tunnel: [w869] -> w858 mode=indexing
                tunnel: w850 -> [w868]
                tunnel: w849 -> [w864]
                n316 = Search 1D Array(1D array=w873, element=w865) -> (index of element=w871:i32)  [unwired: 1 in]
                n317 = Index Array(array=w872, index=w871) -> (element=w866:dbl)
                n318 = case shown="True" w868 {
                  tunnel: [w874 w875] -> w867
                  tunnel: w866 -> [w874 w877]
                  tunnel: w865 -> [_ w889]
                  tunnel: w864 -> [_ w878]
                  frame False {
                  }
                  frame True {
                    n319 = Reverse String(1:w889) -> (0:w888:string)
                    n320 = Match Pattern(string=w888, regular expression="=") -> (before substring=w886:string)  [unwired: 1 in, 3 out]
                    n321 = Reverse String(1:w886) -> (0:w885:string)
                    n322 = Fract/Exp String To Number(string=w885) -> (number=w884:dbl)  [unwired: 3 in, 1 out]
                    n323 = Subtract(x=w884, y=50.0) -> (x-y=w882:dbl)
                    n324 = Divide(x=w882, y=100.0) -> (x/y=w880:dbl)
                    n325 = To Long Integer(number=w880) -> (32bit integer=w879:i32)
                    n326 = Index Array(array=w878, index=w879) -> (element=w876:dbl)
                    n327 = Subtract(x=w877, y=w876) -> (x-y=w875:dbl)
                  }
                }
                n328 = Multiply(x=w867, y=w870) -> (x*y=w869:dbl)
              }
              n329 = Add Array Elements(numeric array=w859) -> (sum=w856:dbl)
              n330 = Add Array Elements(numeric array=w858) -> (sum=w857:dbl)
              n331 = Divide(x=w857, y=w856) -> (x/y=w851:dbl)
              n332 = Replace Array Subset(array=w855, new element=w851, index (row)=w853, index (col)=w852) -> (w854:dbl[][])
            }
            "Temperature" <- w844
            n333 = Array Max & Min(array=w839) -> (max value=w837:dbl, min value=w836:dbl)  [unwired: 2 out]
            n334 = Subtract(x=w837, y=w836) -> (x-y=→"Max Delta T":dbl)
            n335 = Bundle(w837, u32 16721152) -> (w842:cluster{dbl, u32})  [unwired: 1 out]
            n336 = Bundle(w836, u32 3743) -> (w843:cluster{dbl, u32})  [unwired: 1 out]
            n337 = Build Array(w842, w843) -> (w838:cluster{dbl, u32}[])
            n338 = property on="Temperature" class="IntGraph (strict)"("ZScale.MarkerVals[]"=w838) -> ()  [unwired: 2 in, 2 out]
          }
          frame #6 {
            n339 = Array Max & Min(array=w911) -> (max value=w912:dbl)  [unwired: 3 out]
            n340 = for {
              tunnel: w922 -> [w950] mode=indexing
              tunnel: w921 -> [w949]
              tunnel: w920 -> [w948]
              tunnel: w912 -> [w936]
              tunnel: "Kp Lamps" -> [w943]
              tunnel: [w938] -> w916 mode=indexing
              tunnel: [w937] -> w908 mode=indexing
              tunnel: w911 -> [w935] mode=indexing
              tunnel: [w934] -> w910 mode=indexing
              tunnel: [w933] -> w904 mode=indexing
              tunnel: [w932] -> w903 mode=indexing
              tunnel: [w931] -> w892 mode=indexing
              n341 = Unbundle(w950) -> ("Ch Name"=w937:string, w933:i32, w932:i32)  [unwired: 2 out]
              n342 = call "Read_value_of_earlier_Ch.vi"("Desired Ch to Read"=w937, "Ch names"=w948, "Present scan array"=w949) -> ("Value"=w934:dbl, "Scan comment"=w931:string)  [unwired: 1 in]
              n343 = Subtract(x=w936, y=w935) -> (x-y=w942:dbl)
              n344 = Multiply(x=w943, y=w942) -> (x*y=w944:dbl)
              n345 = In Range and Coerce(upper limit=8.0, x=w944, lower limit=-8.0) -> (coerced(x)=w947:dbl)  [unwired: 1 out]
              n346 = Add(x=w934, y=w947) -> (x+y=w939:dbl)
              n347 = Not A Number/Path/Refnum?(number/path/refnum=w939) -> (NaN/Path/Refnum?=w940:bool)
              n348 = Select(t=0.0, s=w940, f=w939) -> (s? t:f=w938:dbl)
            }
            n349 = Array Max & Min(array=w916) -> (min value=w915:dbl)  [unwired: 3 out]
            n350 = Subtract(x=w916, y=w915) -> (x-y=w914:dbl[])
            n351 = In Range and Coerce(upper limit=100.0, x=w914, lower limit=0.0) -> (coerced(x)=w909:dbl[])  [unwired: 1 out]
            n352 = for {
              tunnel: w910 -> [w930] mode=indexing
              tunnel: w909 -> [w923] mode=indexing
              tunnel: [w929] -> w907 mode=indexing if=w928
              tunnel: w908 -> [w929] mode=indexing
              tunnel: [w923] -> w906 mode=indexing if=w928
              shift-right: [w926] -> w896
              shift-left: w905 -> [w927]
              tunnel: w904 -> [w925] mode=indexing
              tunnel: w903 -> [w924] mode=indexing
              n353 = Replace Array Subset(array=w927, new element=w923, index (row)=w925, index (col)=w924) -> (w926:dbl[][])
              n354 = Not Equal?(x=w923, y=w930) -> (x != y?=w928:bool)
            }
            "Power" <- w896
            n355 = Array Max & Min(array=w896) -> (max value=w898:dbl, min value=w897:dbl)  [unwired: 2 out]
            n356 = Bundle(w898, u32 16721152) -> (w901:cluster{dbl, u32})  [unwired: 1 out]
            n357 = Bundle(w897, u32 3743) -> (w902:cluster{dbl, u32})  [unwired: 1 out]
            n358 = Build Array(w901, w902) -> (w895:cluster{dbl, u32}[])
            n359 = property on="Power" class="IntGraph (strict)"("ZScale.MarkerVals[]"=w895) -> ()  [unwired: 2 in, 2 out]
            n360 = call "ASYNC_Adam_server.vi"("Values"=w906, "Channel Names"=w907) -> ("Scan Comments"=w891:string[])  [unwired: 1 in, 2 out]
            n361 = Concatenate Strings(w894, w893, w892, w891) -> (w890:string)
          }
        }
      }
      frame "Check EnFlo tweak factor?" {
        n362 = global read "ADAM_Global.vi" "Client State Array"() -> (w954:T14[])
        n363 = for {
          tunnel: w954 -> [w965] mode=indexing
          tunnel: [w958] -> w952
          stop <- w959 stop-if-true
          n364 = Unbundle By Name(w965) -> ("Client Name"=w961:string, "Traverse level State"=w964:T5)
          n365 = Equal?(x=w964, y=Traverse_Level_State."Running" ("Traverse level State")) -> (x = y?=w958:bool)
          n366 = Equal?(x="EnFlo_Tunnel" ("y"), y=w961) -> (x = y?=w960:bool)
          n367 = And(x=w960, y=w958) -> (x .and. y?=w959:bool)
        }
        n368 = case shown="True" w952 {
          tunnel: ["Lab Temp Control" "Are Inlet Screens Blocked?"] -> w953
          frame False {
          }
          frame True {
          }
        }
      }
      frame "Are Inlet Screens Blocked?" {
        n369 = disable-structure shown="Disabled" {
          frame Disabled {
            n370 = stacked-sequence {
              seq-local: [w969 _] -> [_ w984]
              seq-local: [w972 _] -> [_ w983]
              frame #0 {
                n371 = Build Array("Status:of:EnFlo_Tunnel", "EnFlo_Tunnel:Inlet:K_Factor") -> (w974:string[])
                n372 = call "Get_Channel_averages.vi"("Desired Ch Names"=w974, "Averaging time (mins)"=60.0) -> ("number"=w980:dbl[])  [unwired: 1 in, 2 out]
                n373 = Index Array(array=w980, index=1) -> (element=w969:dbl)
                n374 = Index Array(array=w980, index=0) -> (element=w979:dbl)
                n375 = Greater?(x=w969, y="Max K Factor") -> (0:w971:bool)
                n376 = Equal?(x=w979, y=2.0) -> (x = y?=w977:bool)
                n377 = Compound Arithmetic op=AND(w971, w977) -> (w972:bool)
              }
              frame #1 {
                n378 = case shown="True" w983 {
                  tunnel: w984 -> [_ w988]
                  frame False {
                  }
                  frame True {
                    n379 = Format Into String(format string="The Inlet K factor for the EnFlo Tunnel is now %.2f. This may indicate that the screens need cleaning." ("Format String"), w988) -> (resulting string=w986:string)  [unwired: 2 in, 1 out]
                    n380 = call "Server_Emails.vi"("Client Name Contains"="EnFlo_Tunnel", "Message"=w986, "Subject"="EnFlo Tunnel Screens" ("Message")) -> ()  [unwired: 2 in, 3 out]
                  }
                }
              }
            }
          }
          frame Enabled {
          }
        }
      }
      frame "Lab Temp Control" {
        n381 = call "EnFlo_Lab_Temp_Control.vi"("Current Time"=w991) -> ()
      }
      frame "Is Dew point meter Alive?" {
        n382 = Build Array (concatenate)(w1012, string[] ["EnFlo_Tunnel:Chiller_Pump:Running", "EnFlo_Tunnel:Floor_Cooling:Enable"] ("appended array")) -> (w1011:string[])
        n383 = call "Read_Earlier_Channels.vi"("Present scan array"=w1014, "Ch names"=w1013, "Desired Channels"=w1011) -> ("Scan comments"=w995:string, "Index 0"=w1010:dbl, "Index 1"=w1009:dbl, "Index 2"=w1000:dbl)  [unwired: 2 out]
        n384 = Not A Number/Path/Refnum?(number/path/refnum=w1010) -> (NaN/Path/Refnum?=w1006:bool)
        n385 = Greater?(x=w1000, y=0.5) -> (0:w999:bool)
        n386 = Greater?(x=w1009, y=0.5) -> (0:w1008:bool)
        n387 = while {
          tunnel: [w1019] -> w1004
          tunnel: [w1020] -> w1005
          shift-left: _ -> [w1020]
          tunnel: w1006 -> [w1021]
          shift-left: _ -> [w1019]
          shift-right: [w1021] -> _
          stop <- FALSE continue-if-true
        }
        n388 = Compound Arithmetic op=AND(invert w1006, w1008, w999) -> (w1007:bool)
        n389 = Compound Arithmetic op=AND(w1004, invert w1005, w1006) -> (w1015:bool)
        n390 = case shown="True" w1015 {
          frame False {
          }
          frame True {
            w1022 = TRUE  # Contact All clients?
            n391 = call "Server_Emails.vi"("Message"="The humidity meter is not communicating with the server.\nIt can be reset by switching the toggle switch off and then on again after about 15 seconds." ("Bundle Element"), "Contact All clients?"=w1022, "Subject"="Humidity Meter Offline" ("Error Type")) -> ()  [unwired: 2 in, 3 out]
          }
        }
        n392 = Select(t="Condensation Alert 1", s=w1007, f="More checks") -> (s? t:f=w1017:string)
        n393 = Concatenate Strings(w996, w995) -> (w994:string)
      }
      frame "Condensation Alert 1" {
        w1032 = "EnFlo Lab:Hygrometry:Dew Point temp_PN"
        w1034 = "EnFlo_Tunnel:Chilled Water:Dem Temp"
        n394 = Build Array(w1032, w1034) -> (w1039:string[])
        n395 = while {
          tunnel: [w1047] -> w1035
          tunnel: [w1048] -> w1038
          shift-left: _ -> [w1048]
          shift-right: [w1044] -> w1037
          tunnel: w1039 -> [w1053]
          tunnel: w1040 -> [w1054]
          tunnel: w1041 -> [w1055]
          tunnel: [w1045] -> w1033
          tunnel: [w1044] -> w1031
          tunnel: [w1043] -> w1025 mode=indexing
          stop <- FALSE continue-if-true
          n396 = call "Read_Earlier_Channels.vi"("Present scan array"=w1055, "Ch names"=w1054, "Desired Channels"=w1053) -> ("Scan comments"=w1043:string, "Index 0"=w1047:dbl, "Index 1"=w1045:dbl)  [unwired: 3 out]
          n397 = Select(t=1.5, s=w1048, f=0.5) -> (s? t:f=w1049:dbl)
          n398 = Add(x=w1047, y=w1049) -> (x+y=w1052:dbl)
          n399 = Greater?(x=w1052, y=w1045) -> (0:w1044:bool)
        }
        n400 = Compound Arithmetic op=AND(invert w1038, w1037) -> (w1036:bool)
        n401 = case shown="True" w1036 {
          tunnel: w1035 -> [_ w1059]
          tunnel: w1034 -> [_ w1058]
          tunnel: w1033 -> [_ w1057]
          tunnel: w1032 -> [_ w1056]
          frame False {
          }
          frame True {
            n402 = Format Into String(format string="The %s is %.1f deg C  and the %s is %.1f. \n\nCondensation on the tunnel floor or in the heat exchanger could be occuring." ("Format String"), w1056, w1059, w1058, w1057) -> (resulting string=w1061:string)  [unwired: 2 in, 1 out]
            n403 = call "Server_Emails.vi"("Client Name Contains"="EnFlo_Tunnel", "Message"=w1061, "Subject"="Condensation Alert1" ("Error Type")) -> ()  [unwired: 2 in, 3 out]
          }
        }
        n404 = Select(t="Condensation Alert 2", s=w1031, f="More checks") -> (s? t:f=w1028:string)
        n405 = Concatenate Strings(w1027, w1025) -> (w1026:string)
      }
      frame "Condensation Alert 2" {
        w1068 = "EnFlo Lab:Hygrometry:Dew Point temp_PN"
        w1070 = "EnFlo_Tunnel:Chilled Water:Dem Temp"
        n406 = Build Array(w1068, w1070) -> (w1075:string[])
        n407 = while {
          tunnel: [w1083] -> w1071
          tunnel: [w1084] -> w1074
          shift-left: _ -> [w1084]
          shift-right: [w1080] -> w1073
          tunnel: w1075 -> [w1089]
          tunnel: w1076 -> [w1090]
          tunnel: w1077 -> [w1091]
          tunnel: [w1081] -> w1069
          tunnel: [w1079] -> w1064 mode=indexing
          stop <- FALSE continue-if-true
          n408 = call "Read_Earlier_Channels.vi"("Present scan array"=w1091, "Ch names"=w1090, "Desired Channels"=w1089) -> ("Scan comments"=w1079:string, "Index 0"=w1083:dbl, "Index 1"=w1081:dbl)  [unwired: 3 out]
          n409 = Select(t=0.5, s=w1084, f=-0.5) -> (s? t:f=w1085:dbl)
          n410 = Add(x=w1083, y=w1085) -> (x+y=w1088:dbl)
          n411 = Greater?(x=w1088, y=w1081) -> (0:w1080:bool)
        }
        n412 = Compound Arithmetic op=AND(invert w1074, w1073) -> (w1072:bool)
        n413 = case shown="True" w1072 {
          tunnel: w1071 -> [_ w1095]
          tunnel: w1070 -> [_ w1094]
          tunnel: w1069 -> [_ w1093]
          tunnel: w1068 -> [_ w1092]
          frame False {
          }
          frame True {
            n414 = Format Into String(format string="The %s is %.1f deg C  and the %s is %.1f. \n\nCondensation on the tunnel floor or in the heat exchanger could well be occuring." ("Format String"), w1092, w1095, w1094, w1093) -> (resulting string=w1097:string)  [unwired: 2 in, 1 out]
            n415 = call "Server_Emails.vi"("Client Name Contains"="EnFlo_Tunnel", "Message"=w1097, "Subject"="Condensation Alert2" ("Error Type")) -> ()  [unwired: 2 in, 3 out]
          }
        }
        n416 = Concatenate Strings(w1066, w1064) -> (w1065:string)
      }
      frame "More checks" {
        n417 = Build Array("EnFlo_Tunnel:Gas Solenoid:Status", "GMU:Gas:Enable") -> (w1115:string[])
        n418 = call "Read_Earlier_Channels.vi"("Present scan array"=w1117, "Ch names"=w1116, "Desired Channels"=w1115) -> ("Scan comments"=w1114:string, "Index 0"=w1102:dbl, "Index 1"=w1101:dbl)  [unwired: 3 out]
        n419 = Greater?(x=w1101, y=0.5) -> (0:w1107:bool)
        n420 = Less?(x=w1102, y=0.5) -> (x < y?=w1106:bool)
        n421 = And(x=w1106, y=w1107) -> (x .and. y?=w1105:bool)
        n422 = feedback-in #6(w1105) -> ()
        n423 = feedback #6() -> (w1104:bool)  [unwired: 1 in]
        n424 = Compound Arithmetic op=AND(w1105, invert w1104) -> (w1103:bool)
        n425 = case shown="True" w1103 {
          frame False {
          }
          frame True {
            w1119 = TRUE  # Contact All clients?
            n426 = call "Server_Emails.vi"("Message"="The GMU:Gas:Enable is on but the  EnFlo_Tunnel:Gas Solenoid:Status is off. The IR2100 detector is showing a gas concentration that is above the Lower Explosive Limit." ("Bundle Element"), "Contact All clients?"=w1119, "Subject"="Gas Solenoid:Status" ("Error Type")) -> ()  [unwired: 2 in, 3 out]
          }
        }
        n427 = Concatenate Strings(w1113, w1114) -> (w1112:string)
      }
      frame "End" {
        n428 = stacked-sequence {
          seq-local: [w1149 _] -> [_ w1179]
          seq-local: [w1146 _] -> [_ w1176]
          seq-local: [w1131 _] -> [_ w1175]
          tunnel: w1129 -> [w1153 _]
          tunnel: w1128 -> [w1141 w1178]
          tunnel: w1127 -> [w1142 w1177]
          tunnel: w1126 -> [_ _]
          tunnel: [w1137 _] -> w1124
          frame #0 {
            n429 = call <vilib>:"LV70TimeStampToDateRec.vi"("time stamp"=w1153) -> ("date time rec"=w1154:T15)
            n430 = Unbundle By Name(w1154) -> ("hour"=w1152:i32, "day of week"=w1132:i32, "minute"=w1145:i32, "day of year"=w1131:i32)
            n431 = Less?(x=w1145, y=3) -> (x < y?=w1143:bool)
            n432 = while {
              tunnel: w1152 -> [w1161]
              tunnel: w1132 -> [w1174]
              shift-right: [w1170] -> w1150
              shift-left: _ -> [w1169]
              tunnel: [w1169] -> w1151
              tunnel: w1143 -> [w1167]
              stop <- FALSE continue-if-true
              n433 = Equal?(x=w1161, y=16) -> (x = y?=w1156:bool)
              n434 = Equal?(x=w1161, y=12) -> (x = y?=w1158:bool)
              n435 = Equal?(x=w1161, y=14) -> (x = y?=w1157:bool)
              n436 = Equal?(x=w1161, y=8) -> (x = y?=w1160:bool)
              n437 = Equal?(x=w1161, y=10) -> (x = y?=w1159:bool)
              n438 = In Range and Coerce(upper limit=7, x=w1174, lower limit=1) -> (In Range?=w1171:bool)  [unwired: 1 out]
              n439 = Compound Arithmetic op=OR(w1160, w1159, w1158, w1157, w1156) -> (w1155:bool)
              n440 = Compound Arithmetic op=AND(w1155, w1171, w1167) -> (w1170:bool)
            }
            n441 = call "Read_value_of_earlier_Ch.vi"("Desired Ch to Read"="Uni:Chilled Water:Temp", "Ch names"=w1141, "Present scan array"=w1142) -> ("Value"=w1146:dbl, "Scan comment"=w1139:string)  [unwired: 1 in]
            n442 = call "Read_value_of_earlier_Ch.vi"("Desired Ch to Read"="EnFlo_Lab:Shut:Down", "Ch names"=w1141, "Present scan array"=w1142) -> ("Value"=w1136:dbl, "Scan comment"=w1138:string)  [unwired: 1 in]
            n443 = Greater?(x=w1146, y=12.0) -> (0:w1134:bool)
            n444 = Less?(x=w1136, y=0.5) -> (x < y?=w1133:bool)
            n445 = Compound Arithmetic op=AND(w1134, w1133, invert w1151, w1150) -> (w1149:bool)
            n446 = Concatenate Strings(w1139, w1138) -> (w1137:string)
          }
          frame #1 {
            n447 = case shown="True" w1179 {
              tunnel: w1178 -> [_ _]
              tunnel: w1177 -> [_ _]
              tunnel: w1176 -> [_ w1183]
              tunnel: w1175 -> [_ w1180]
              frame False {
              }
              frame True {
                n448 = feedback-in #7(w1180) -> ()
                n449 = feedback #7() -> (w1181:i32)  [unwired: 1 in]
                n450 = Not Equal?(x=w1181, y=w1180) -> (x != y?=w1182:bool)
                n451 = case shown="True" w1182 {
                  tunnel: w1183 -> [_ w1191]
                  frame False {
                  }
                  frame True {
                    n452 = Select(t=string[] [], s="Disable Sending email to estates regarding Chilled water Temp", f=string[] ["efmenquiries@surrey.ac.uk"] ("Extra People to Email")) -> (s? t:f=w1184:string[])
                    n453 = Format Into String(format string="\n\nDear Estates\n\nThe monitoring system in the EnFlo Lab (01AB01) is currently indicating that the Chilled water in the AB Building is at %.0f deg C.\n\nPlease could you arrange for somebody to come and investigate this please.\n\nThanks very much\n\nPaul Hayden x9545  or Mobile  07961 608409", w1191) -> (resulting string=w1190:string)  [unwired: 2 in, 1 out]
                    n454 = call "Server_Emails.vi"("Message"=w1190, "Contact All clients?"=TRUE, "Subject"="Chilled water in AB Building above 12 deg C" ("Error Type"), "Extra People to Email"=w1184) -> ()  [unwired: 1 in, 3 out]
                  }
                }
              }
            }
          }
        }
        n455 = Concatenate Strings(w1123, w1124) -> (w1122:string)
      }
      frame "No Match", Default {
        n456 = Current VI's Path() -> (path=w1197:path)
        n457 = Format Into String(format string="The Case\"%s\" was not Matched\nin VI named\n'%s\"" ("Format String"), w1196, w1197) -> (resulting string=w1200:string)  [unwired: 2 in, 1 out]
        n458 = One Button Dialog(message=w1200, button name ("OK")="STOP") -> (true=w1198:bool)
        n459 = Stop(stop? (T)=w1198) -> ()
      }
    }
  }
  "Scan Comments" <- w1
